vi "Calibration Main.vi"(8 "error in (no error)":errorcluster, 11 "Pump Calibration Config in":T1={"Settings"={"Cycle Period"=500.0, "Ismatech"={"VISA resource name"="", "Simulated?"=TRUE, "Pump Number"=1.0, "Reverse?"=FALSE}, "Masterflex"={"VISA resource name"="", "Simulated?"=TRUE, "Pump Number"=1.0, "Reverse?"=FALSE}, "Bronkhorst M13 Settings"={"VISA resource name"="", "Simulated?"=TRUE, "Smoothing Steps"=1}, "PID 2 Parameters"={"Input Device"=enum."Default", "Output Device"=enum."Default"}, "Tacmina Settings"={"Analog DAQ Task"="", "Digital DAQ Task"=""}, "KNF SIMDOS Settings"={"VISA resource name"="", "Simulated?"=TRUE}, "VICI M50 Settings"={"VISA resource name"="", "Pump ID"="", "Pump Head Vol"=0.0, "Reverse?"=FALSE, "Simulated?"=TRUE}, "FLOM Settings"={"VISA resource name"="", "Simulated?"=TRUE, "Pump Number"=0.0}, "Calibration Limits"={"Minimum (ml/min)"=0.0, "Maximum (ml/min)"=0.0, "Steps"=0.0}, "SSI PR Settings"={"VISA resource name"="", "Simulated?"=FALSE}, "Ismatech 4308 Settings"={"VISA resource name"="", "Pump Number"=1, "Channel Number"=0, "Simulated?"=TRUE, "Reverse?"=FALSE}, "Bronkhorst M14 Settings"={"VISA resource name"="", "Simulated?"=FALSE, "Smoothing Steps"=1}}, "Flowmeter Output"=0.0, "Density"=0.0, "FL Temp"=0.0, "Speed %"=0.0, "File Refnum"=refnum, "Pump On?"=enum."Not Initialized"} {"Settings"."Bronkhorst M14 Settings"."Smoothing Steps" min=1 step=1; "Settings"."Ismatech 4308 Settings"."Channel Number" min=0 max=3; "Settings"."Ismatech 4308 Settings"."Pump Number" min=1; "Settings"."Bronkhorst M13 Settings"."Smoothing Steps" min=1 step=1; "Settings"."Masterflex"."Pump Number" min=1.0 max=20.0 step=1.0; "Settings"."Ismatech"."Pump Number" min=1.0 max=20.0 step=1.0}) -> (0 "error out":errorcluster, 3 "Pump Calibration Config out":T1={"Settings"={"Cycle Period"=500.0, "Ismatech"={"VISA resource name"="", "Simulated?"=TRUE, "Pump Number"=1.0, "Reverse?"=FALSE}, "Masterflex"={"VISA resource name"="", "Simulated?"=TRUE, "Pump Number"=1.0, "Reverse?"=FALSE}, "Bronkhorst M13 Settings"={"VISA resource name"="", "Simulated?"=TRUE, "Smoothing Steps"=1}, "PID 2 Parameters"={"Input Device"=enum."Default", "Output Device"=enum."Default"}, "Tacmina Settings"={"Analog DAQ Task"="", "Digital DAQ Task"=""}, "KNF SIMDOS Settings"={"VISA resource name"="", "Simulated?"=TRUE}, "VICI M50 Settings"={"VISA resource name"="", "Pump ID"="", "Pump Head Vol"=0.0, "Reverse?"=FALSE, "Simulated?"=TRUE}, "FLOM Settings"={"VISA resource name"="", "Simulated?"=TRUE, "Pump Number"=0.0}, "Calibration Limits"={"Minimum (ml/min)"=0.0, "Maximum (ml/min)"=0.0, "Steps"=0.0}, "SSI PR Settings"={"VISA resource name"="", "Simulated?"=FALSE}, "Ismatech 4308 Settings"={"VISA resource name"="", "Pump Number"=1, "Channel Number"=0, "Simulated?"=TRUE, "Reverse?"=FALSE}, "Bronkhorst M14 Settings"={"VISA resource name"="", "Simulated?"=FALSE, "Smoothing Steps"=1}}, "Flowmeter Output"=0.0, "Density"=0.0, "FL Temp"=0.0, "Speed %"=0.0, "File Refnum"=refnum, "Pump On?"=enum."Not Initialized"} {"Settings"."Bronkhorst M14 Settings"."Smoothing Steps" min=1 step=1; "Settings"."Ismatech 4308 Settings"."Channel Number" min=0 max=3; "Settings"."Ismatech 4308 Settings"."Pump Number" min=1; "Settings"."Bronkhorst M13 Settings"."Smoothing Steps" min=1 step=1; "Settings"."Masterflex"."Pump Number" min=1.0 max=20.0 step=1.0; "Settings"."Ismatech"."Pump Number" min=1.0 max=20.0 step=1.0})   [LabVIEW 2018, in "Calibration.lvlib"]
uses:
  Pfizer Timed Seq/Software/Calibration VIs/Calibration.lvlib
  Pump Calibration Config.ctl
  Pfizer Timed Seq/Software/Ismatec ISM 831C/Controls/Ismatech ISM831C Settings Cluster.ctl
  Pfizer Timed Seq/Software/Masterflex 7550-30/Controls/Settings Cluster.ctl
  Pfizer Timed Seq/Software/Bronkhorst M13 Flow Meter/Settings Cluster.ctl
  Pfizer Timed Seq/Software/Measure Instrument/PID Input Enum.ctl
  Pfizer Timed Seq/Software/Measure Instrument/PID 2 Output Enum.ctl
  Pfizer Timed Seq/Software/Tacmina QI/Tacmina QI DAQ Setting.ctl
  Pfizer Timed Seq/Software/KNF Pump/Settings Cluster plus SIMDOS.ctl
  Pfizer Timed Seq/Software/VICI M50 Party Mode/Settings Cluster.ctl
  Pfizer Timed Seq/Software/FLOM Pump/Settings Cluster.ctl
  Pfizer Timed Seq/Software/SSI PR Class/SSI PR or LD Settings Cluster.ctl
  Pfizer Timed Seq/Software/Ismatec 78001/Ismatec 4083.ctl
  Pfizer Timed Seq/Software/Bronkhorst M14 Flow Meter/Settings Cluster.ctl
  Pfizer Timed Seq/Software/Mettler Toledo/Controls/Settings Cluster.ctl
  Pfizer Timed Seq/Software/ASIA Pump/Pump Settings.ctl
  Pfizer Timed Seq/Software/Masterflex 75211/Masterflex 75211 DAQ Setting.ctl
  <vilib>/Platform/TimedLoop/XDataNode/timing_clust.ctl
  <vilib>/Platform/TimedLoop/XDataNode/nitl_modes.ctl
  <vilib>/Platform/TimedLoop/XDataNode/wakeup.ctl
  Pfizer Timed Seq/Software/support/Message Queue/Enqueue Message (Single).vi
  <vilib>/Utility/file.llb/Read Delimited Spreadsheet (string).vi
  <vilib>/Utility/file.llb/Write Delimited Spreadsheet (string).vi
  <vilib>/Platform/TimedLoop/XDataNode/XDataNode.xnode
  <vilib>/regexp/Match Regular Expression.xnode
  Pfizer Timed Seq/Software/KNF Pump/KNF SIMDOS.lvlib
  Pfizer Timed Seq/Software/Ismatec ISM 831C/Ismatec ISM 831C.lvlib
  Pfizer Timed Seq/Software/VICI M50 Party Mode/VICI M6 M50 Party Mode.lvlib
  Pfizer Timed Seq/Software/Masterflex 7550-30/Masterflex 7550-30.lvlib
  Pfizer Timed Seq/Software/FLOM Pump/FLOM Pump.lvlib
  Pfizer Timed Seq/Software/Bronkhorst M13 Flow Meter/Bronkhorst M13 Flow Meter.lvlib
  Pfizer Timed Seq/Software/Bronkhorst M14 Flow Meter/Bronkhorst M14 Flow Meter.lvlib
  Pfizer Timed Seq/Software/support/Message Queue/Message Queue.lvlib
  Pfizer Timed Seq/Software/SSI PR Class/SSI PR or LD Pump.lvlib
  Support/Engine.lvlib
  <vilib>/Analysis/NI_AALPro.lvlib
  <vilib>/Platform/TimedLoop/XDataNode/XDNodeRunTimeDep.lvlib
  Pfizer Timed Seq/Software/Ismatec 78001/Ismatec 4308.lvlib
  Pfizer Timed Seq/Software/Report Generation/Report Generation.lvlib
  Pfizer Timed Seq/Software/Mettler Toledo/Mettler Toledo.lvlib
  Pfizer Timed Seq/Software/Tacmina QI/Tacmina QI.lvlib
  Pfizer Timed Seq/Software/ASIA Pump.lvlib
  Pfizer Timed Seq/Software/Masterflex 75211/Masterflex 75211.lvlib
panel:
  out "Channel Number":i16
  out "Pump Number":i16
  out "Not Empty":bool
  out "All Good":bool
  out "Y array":dbl[](array[numeric])
  out "X array":dbl[](array[numeric])
  out "Output Selected":bool
  out "Input Selected":bool
  out "Step Array":dbl[](array[numeric])
  in  "?":enum32{"Settings", "Results"}(tab)
  in  "Settings Dialog":T17={"Cycle Period"=500.0, "Ismatech"={"VISA resource name"="", "Simulated?"=FALSE, "Pump Number"=1.0, "Reverse?"=FALSE}, "Masterflex"={"VISA resource name"="", "Simulated?"=FALSE, "Pump Number"=1.0, "Reverse?"=FALSE}, "Mettler"={"VISA resource name"="", "Simulated?"=FALSE}, "Bronkhorst M13 Flow Meter"={"VISA resource name"="", "Simulated?"=FALSE, "Smoothing Steps"=1}, "Setup Parameters"={"Input Device"=enum."Default", "Output Device"=enum."Default"}, "Bronkhorst M14 Settings"={"VISA resource name"="", "Simulated?"=FALSE, "Smoothing Steps"=1}, "Tacmina Settings"={"Analog DAQ Task"="", "Digital DAQ Task"=""}, "KNF SIMDOS Settings"={"VISA resource name"="", "Simulated?"=FALSE}, "ASIA Pump C"={"ASIA Pump #"=-1, "channel"=-1, "Simulated"=FALSE}, "VICI M50 Settings"={"VISA resource name"="", "Pump ID"="", "Pump Head Vol"=0.0, "Reverse?"=FALSE, "Simulated?"=FALSE}, "FLOM Settings"={"VISA resource name"="", "Simulated?"=FALSE, "Pump Number"=1.0}, "Calibration Limits"={"Minimum (ml/min)"=0.0, "Maximum (ml/min)"=0.0, "Steps"=0.0}, "File Name"="", "SSI PR Settings"={"VISA resource name"="", "Simulated?"=FALSE}, "Masterflex 75211 Settings"={"Analog DAQ Task"="", "Digital DAQ Task"=""}, "Ismatech 4308 Settings"={"VISA resource name"="", "Pump Number"=0, "Channel Number"=0, "Simulated?"=FALSE, "Reverse?"=FALSE}} {"Ismatech 4308 Settings"."Channel Number" min=0 max=3; "Ismatech 4308 Settings"."Pump Number" min=1; "Calibration Limits"."Maximum (ml/min)" max=16.5; "ASIA Pump C"."channel" min=-1 max=1 step=1; "Bronkhorst M14 Settings"."Smoothing Steps" min=1 step=1; "Bronkhorst M13 Flow Meter"."Smoothing Steps" min=1 step=1; "Masterflex"."Pump Number" min=1.0 max=20.0 step=1.0; "Ismatech"."Pump Number" min=1.0 max=20.0 step=1.0}
  in  "Start Button":bool
  in  "Cancel Button":bool
  out "Y Intercept":dbl
  in  "Accept Button":bool
  in  "Decline Button":bool
  out "Calibration Graph":cluster{dbl[], dbl[]}[](graph)
  out "Calibration Slope":dbl
  out "R^2 Value":dbl format="%#.4g"
  out "Pump Status":enum16{"Off", "On", "Not Initialized"}(ring)
  # "Output Instruments"
  # "Input Instruments"
  # "Output Instruments"
  # "Input Instruments"
  # "Output Instruments"
  # "Input Instruments"
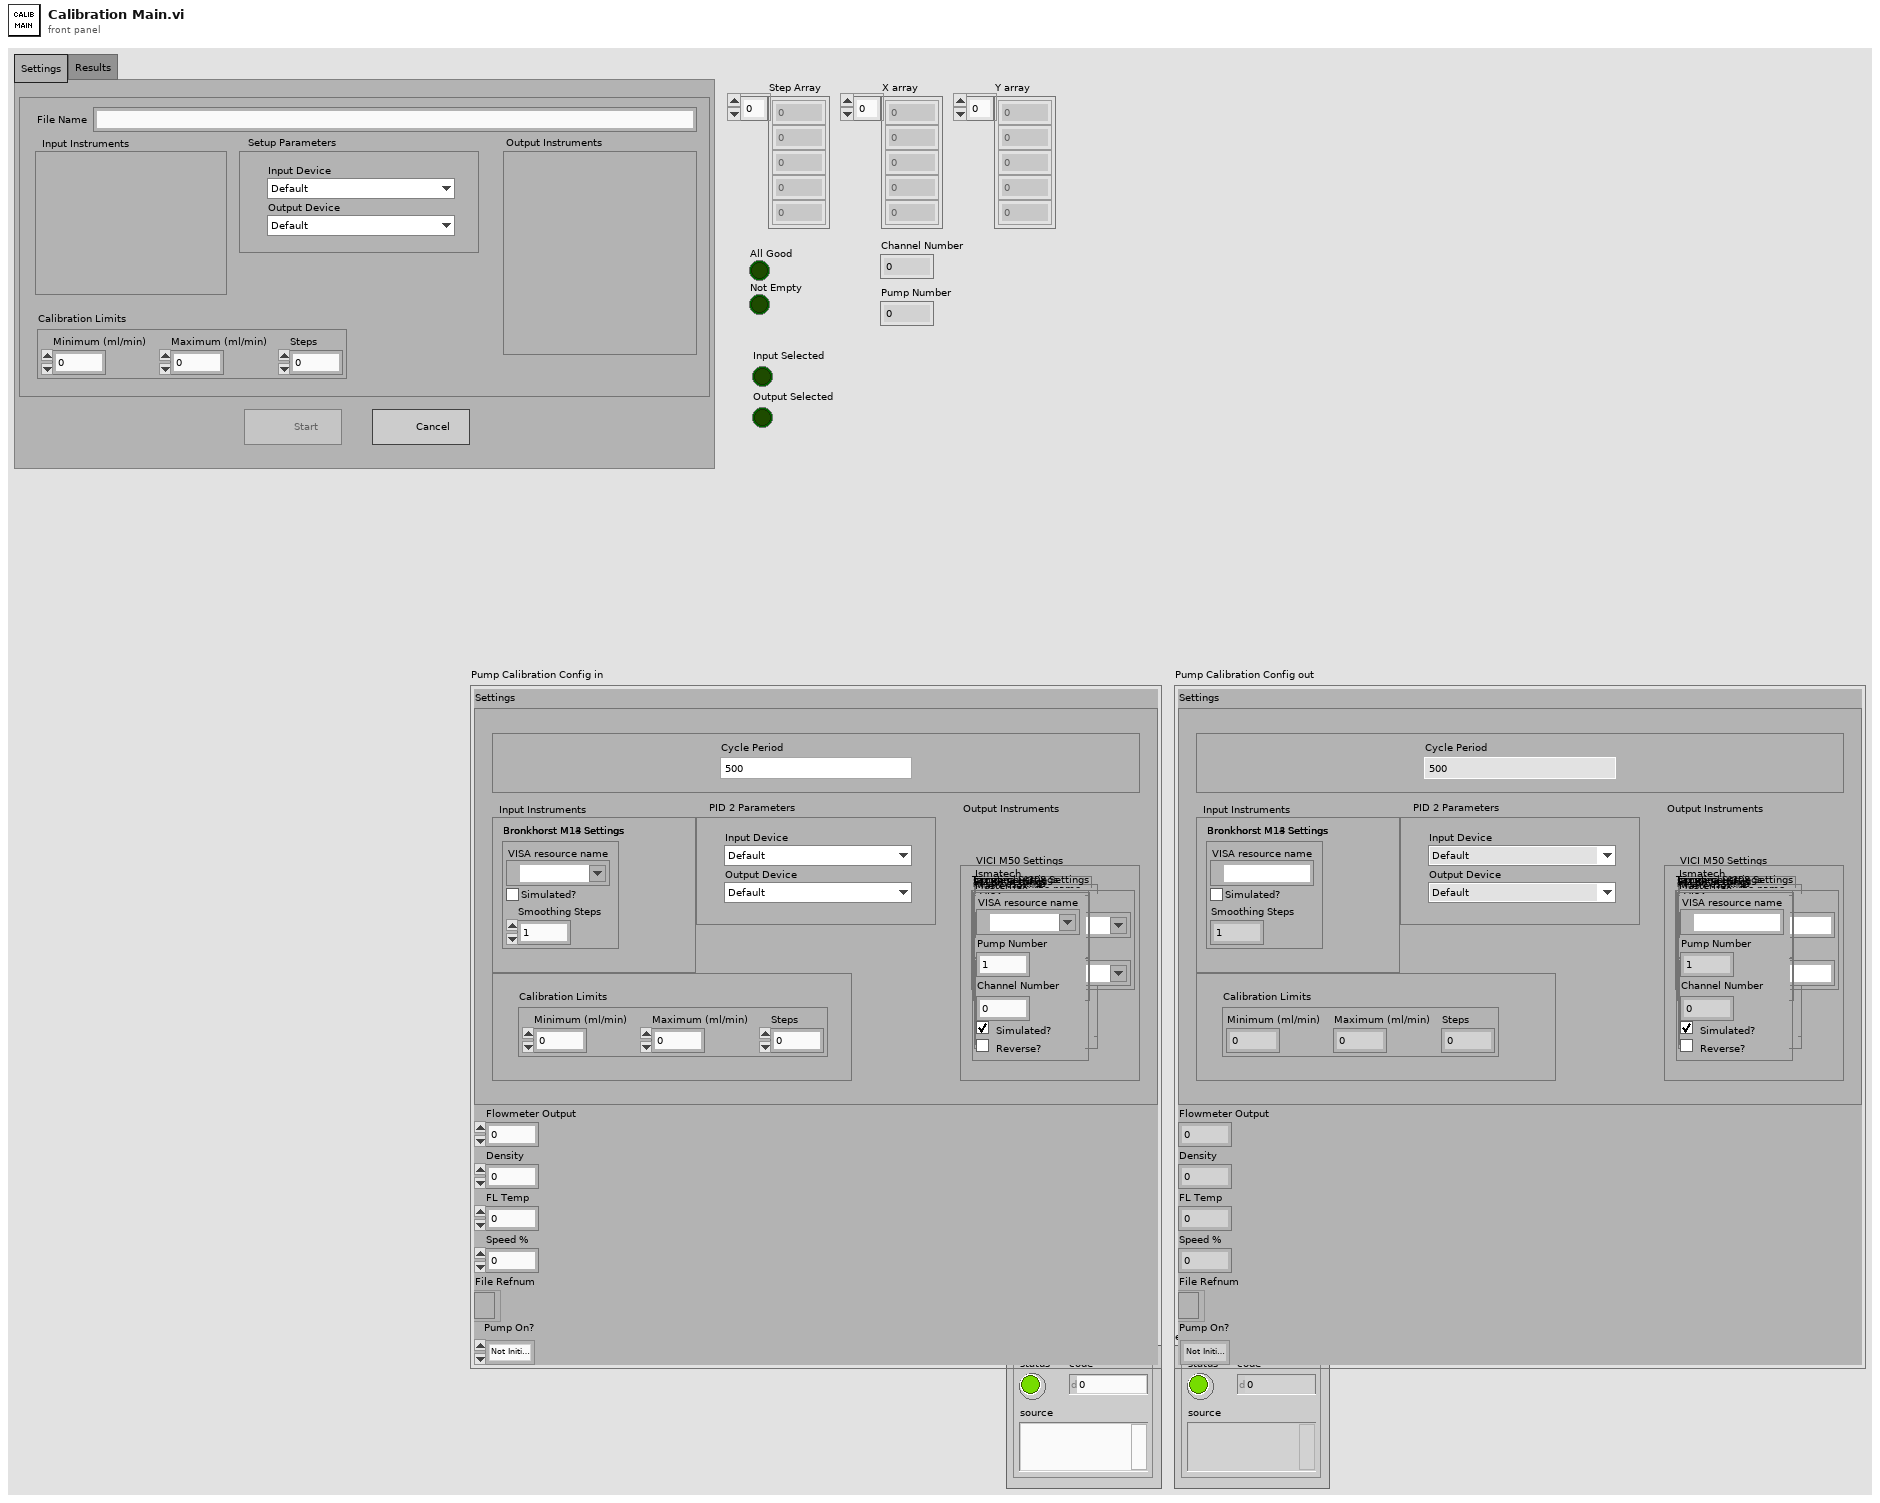
[diagram p1: front panel]
types:
  T1 = typedef "Calibration.lvlib/Pump Calibration Config.ctl" = cluster{"Settings":cluster{"Cycle Period":dbl, "Ismatech":T2, "Masterflex":T3, "Bronkhorst M13 Settings":T4, "PID 2 Parameters":cluster{"Input Device":T5, "Output Device":T6}, "Tacmina Settings":T7, "KNF SIMDOS Settings":T8, "VICI M50 Settings":T9, "FLOM Settings":T10, "Calibration Limits":cluster{"Minimum (ml/min)":dbl, "Maximum (ml/min)":dbl, "Steps":dbl}, "SSI PR Settings":T11, "Ismatech 4308 Settings":T12, "Bronkhorst M14 Settings":T13}, "Flowmeter Output":dbl, "Density":dbl, "FL Temp":dbl, "Speed %":dbl, "File Refnum":refnum<file>, "Pump On?":enum16{"Off", "On", "Not Initialized"}}
  T2 = typedef "Ismatec ISM 831C.lvlib/Ismatech ISM831C Settings Cluster.ctl" = cluster{"VISA resource name":refnum<visa-resource-name>, "Simulated?":bool, "Pump Number":dbl, "Reverse?":bool}
  T3 = typedef "Masterflex 7550-30.lvlib/Settings Cluster.ctl" = cluster{"VISA resource name":refnum<visa-resource-name>, "Simulated?":bool, "Pump Number":dbl, "Reverse?":bool}
  T4 = typedef "Bronkhorst M13 Flow Meter.lvlib/Settings Cluster.ctl" = cluster{"VISA resource name":refnum<visa-resource-name>, "Simulated?":bool, "Smoothing Steps":i32}
  T5 = typedef "PID Input Enum.ctl" = enum16{"Default", "Bronkhorst M13", "Bronkhorst M14", "Scale Rate of Change"}
  T6 = typedef "PID 2 Output Enum.ctl" = enum16{"Default", "Ismatec ISM 4308", "Ismatec ISM 831C", "Masterflex 7550-30", "VICI M6", "VICI M50", "Tacmina QI", "KNF SIMDOS", "ASIA Type C", "FLOM UI-22-11", "SSI PR/LD", "SSI P40", "Masterflex 75211-70"}
  T7 = typedef "Tacmina QI.lvlib/Tacmina QI DAQ Setting.ctl" = cluster{"Analog DAQ Task":refnum<k21>, "Digital DAQ Task":refnum<k21>}
  T8 = typedef "KNF SIMDOS.lvlib/Settings Cluster plus SIMDOS.ctl" = cluster{"VISA resource name":refnum<visa-resource-name>, "Simulated?":bool}
  T9 = typedef "VICI M6 M50 Party Mode.lvlib/Settings Cluster.ctl" = cluster{"VISA resource name":refnum<visa-resource-name>, "Pump ID":string, "Pump Head Vol":dbl, "Reverse?":bool, "Simulated?":bool}
  T10 = typedef "FLOM Pump.lvlib/Settings Cluster.ctl" = cluster{"VISA resource name":refnum<visa-resource-name>, "Simulated?":bool, "Pump Number":dbl}
  T11 = typedef "SSI PR or LD Pump.lvlib/SSI PR or LD Settings Cluster.ctl" = cluster{"VISA resource name":refnum<visa-resource-name>, "Simulated?":bool}
  T12 = typedef "Ismatec 4308.lvlib/Ismatec 4083.ctl" = cluster{"VISA resource name":refnum<visa-resource-name>, "Pump Number":i16, "Channel Number":i16, "Simulated?":bool, "Reverse?":bool}
  T13 = typedef "Bronkhorst M14 Flow Meter.lvlib/Settings Cluster.ctl" = cluster{"VISA resource name":refnum<visa-resource-name>, "Simulated?":bool, "Smoothing Steps":i32}
  T14 = typedef "Mettler Toledo.lvlib/Settings Cluster.ctl" = cluster{"VISA resource name":refnum<visa-resource-name>, "Simulated?":bool}
  T15 = typedef "ASIA Pump.lvlib/Pump Settings.ctl" = cluster{"ASIA Pump #":i32, "channel":i32, "Simulated":bool}
  T16 = typedef "Masterflex 75211.lvlib/Masterflex 75211 DAQ Setting.ctl" = cluster{"Analog DAQ Task":refnum<k21>, "Digital DAQ Task":refnum<k21>}
  T17 = cluster{"Cycle Period":dbl, "Ismatech":T2, "Masterflex":T3, "Mettler":T14, "Bronkhorst M13 Flow Meter":T4, "Setup Parameters":cluster{"Input Device":T5, "Output Device":T6}, "Bronkhorst M14 Settings":T13, "Tacmina Settings":T7, "KNF SIMDOS Settings":T8, "ASIA Pump C":T15, "VICI M50 Settings":T9, "FLOM Settings":T10, "Calibration Limits":cluster{"Minimum (ml/min)":dbl, "Maximum (ml/min)":dbl, "Steps":dbl}, "File Name":string, "SSI PR Settings":T11, "Masterflex 75211 Settings":T16, "Ismatech 4308 Settings":T12}
  T18 = enum8{"Enabled", "Disabled", "Disabled and Grayed Out"}
  T19 = cluster{"Calibration UI":refnum<queue>, "Calibration Engine":refnum<queue>}
  T20 = typedef "XDNodeRunTimeDep.lvlib/timing_clust.ctl" = cluster{"Expected End [f-1]":u64, "Actual End [f-1]":u64, "Finished Late? [f-1]":bool, "Expected End [i-1]":u64, "Actual End [i-1]":u64, "Finished Late? [i-1]":bool, "Expected Start [i]":u64, "Actual Start [i]":u64, "Expected Start [f]":u64, "Actual Start [f]":u64, "Source Name":string, "Structure Name":string, "Period":i64, "Deadline":i64, "Offset":i64, "Start":i64, "Priority":i32, "Timeout":i32, "Mode":T21, "Wakeup Reason":T22, "Error":errorcluster, "Source Type":string, "Secondary Source Type":string, "Global End Time":u64, "Global Start Time":u64, "Frame Duration":u64, "Iteration Duration":u64, "Assigned CPU":i32, "I/O Scan Engine Mode":u32}
  T21 = typedef "XDNodeRunTimeDep.lvlib/nitl_modes.ctl" = enum32{"No Change", "Process missed periods, maintain original phase", "Discard missed periods, maintain original phase", "Process missed periods, ignore original phase", "Discard missed periods, ignore original phase"}
  T22 = typedef "XDNodeRunTimeDep.lvlib/wakeup.ctl" = enum32{"Normal", "Aborted", "Asynchronous wakeup", "Timing source error", "Timed loop error", "Timeout"}
  T23 = enum16{"open", "replace", "create", "open or create", "replace or create", "replace or create with confirmation"}
  T24 = cluster{"R^2":dbl, "Calibration Slope":dbl, "Y Intercept":dbl}
  T25 = cluster{"slope min":dbl, "slope max":dbl, "intercept min":dbl, "intercept max":dbl}
  T26 = cluster{"Minimum (ml/min)":dbl, "Maximum (ml/min)":dbl, "Steps":dbl}
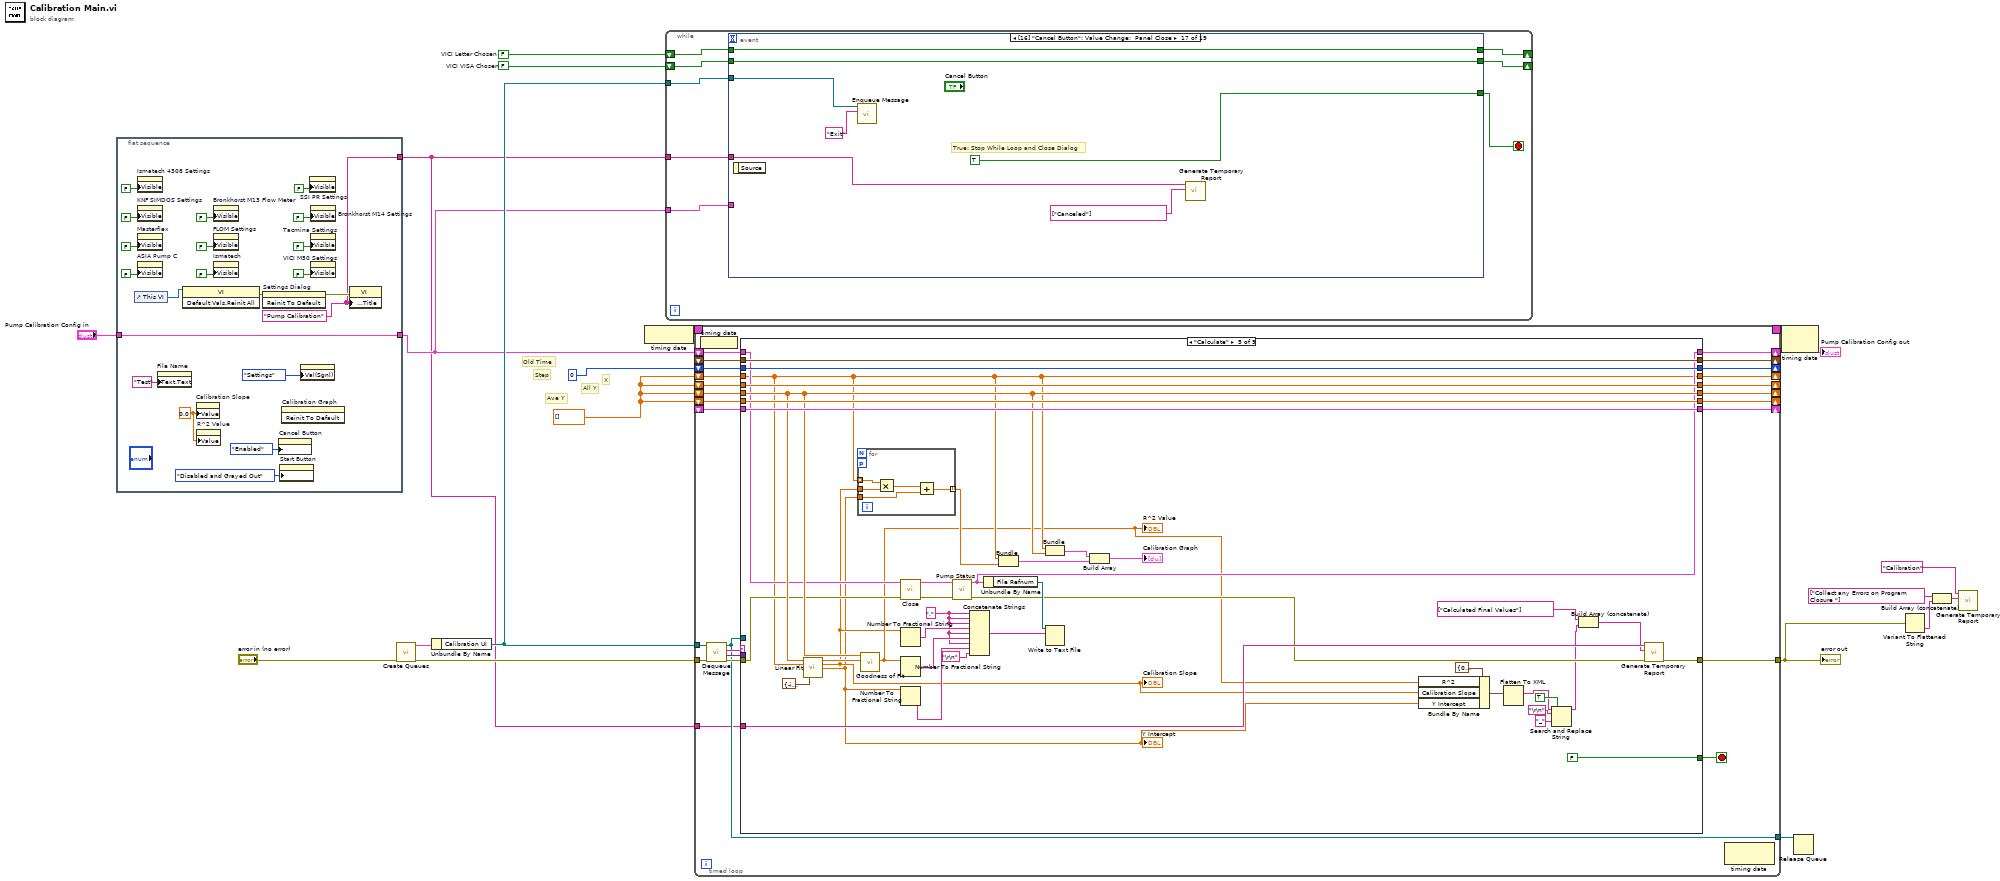
[diagram p0: block diagram]
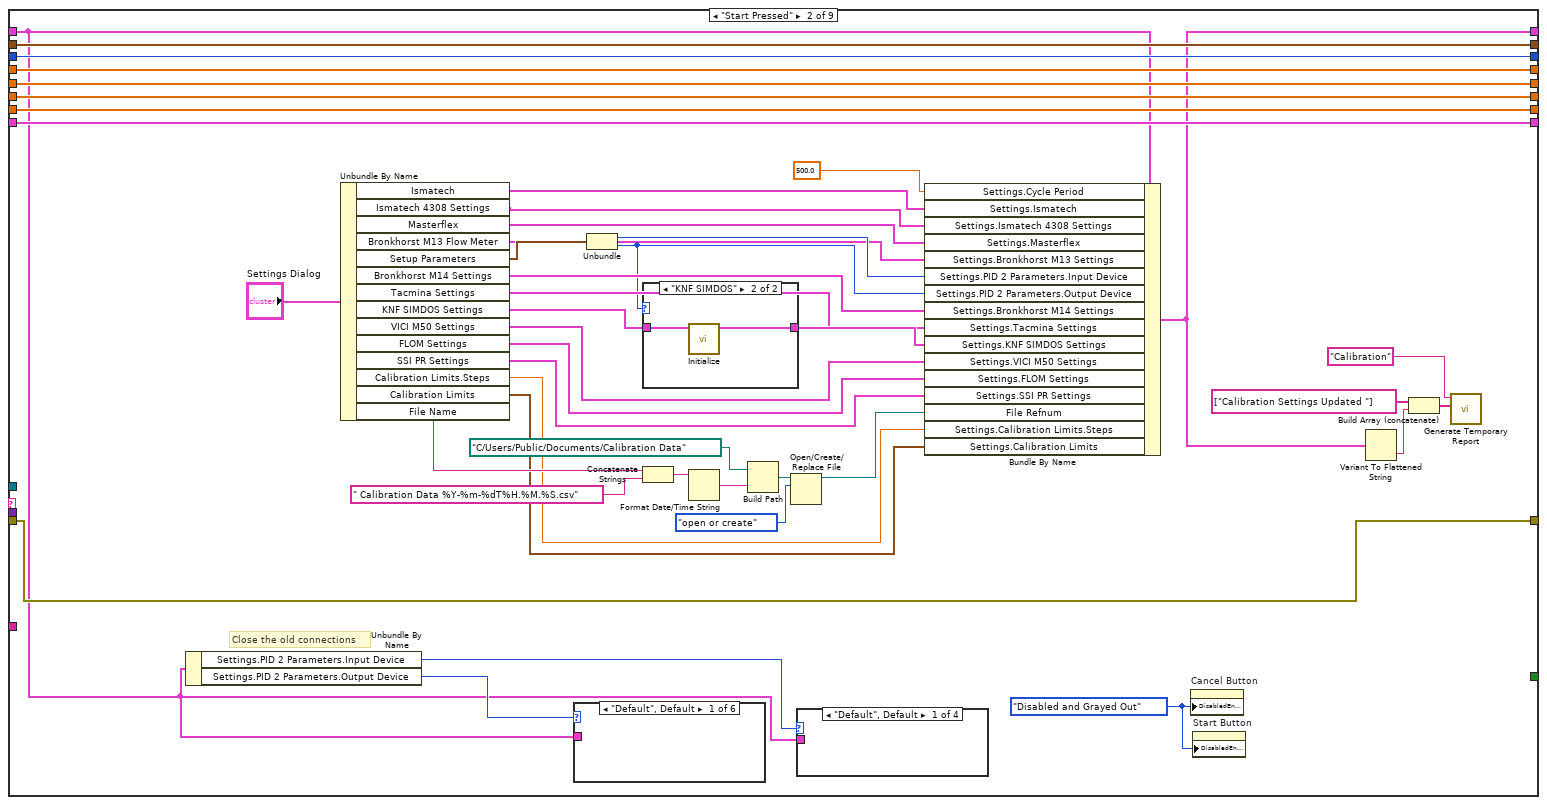
[diagram p3: hidden frame]
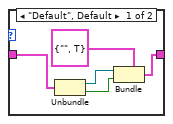
[diagram p4: hidden frame]
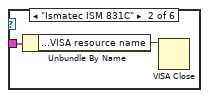
[diagram p5: hidden frame]
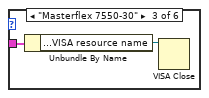
[diagram p6: hidden frame]
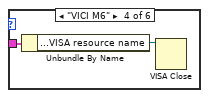
[diagram p7: hidden frame]
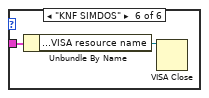
[diagram p9: hidden frame]
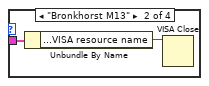
[diagram p10: hidden frame]
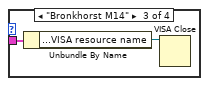
[diagram p11: hidden frame]
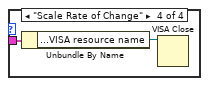
[diagram p12: hidden frame]
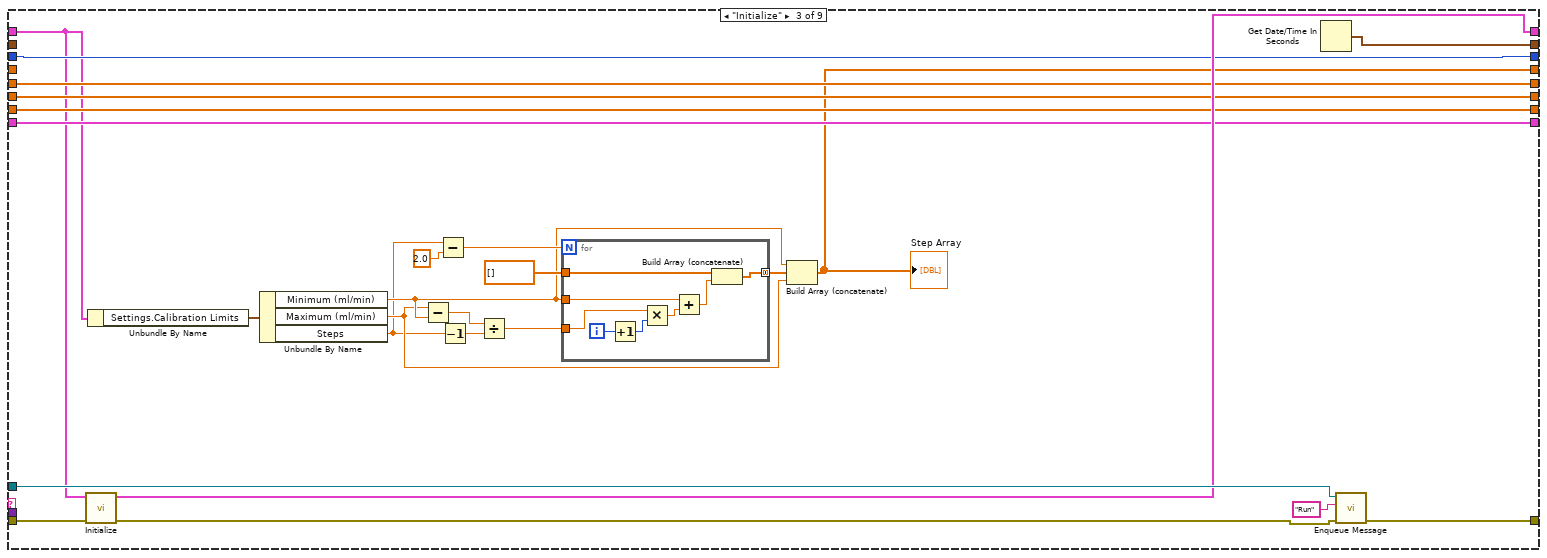
[diagram p13: hidden frame]
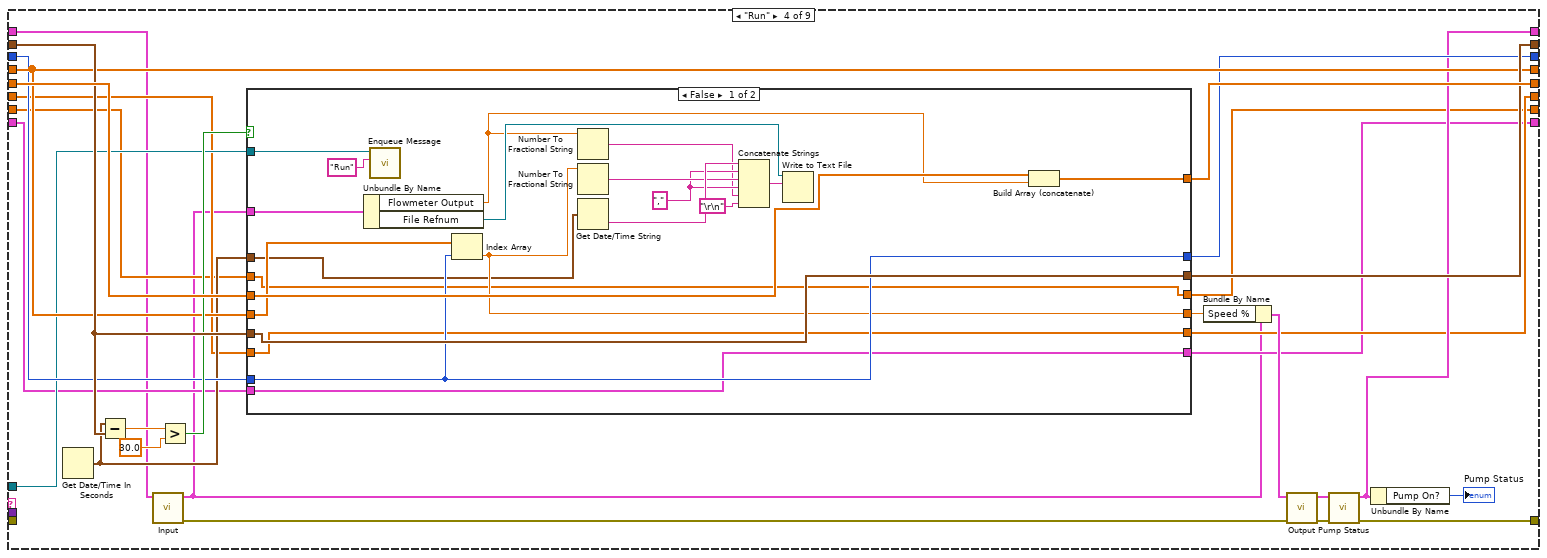
[diagram p14: hidden frame]
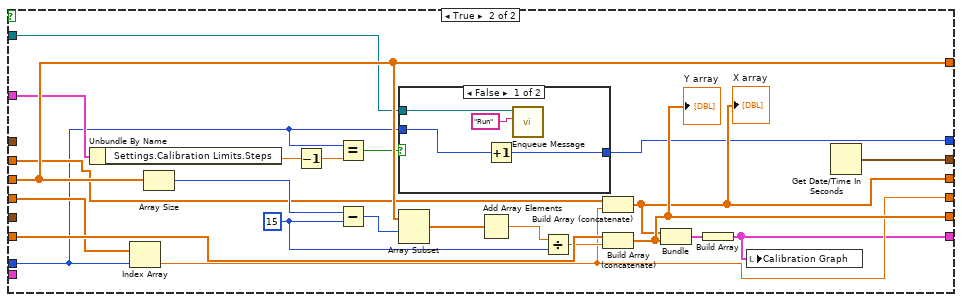
[diagram p15: hidden frame]
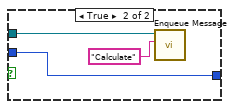
[diagram p16: hidden frame]
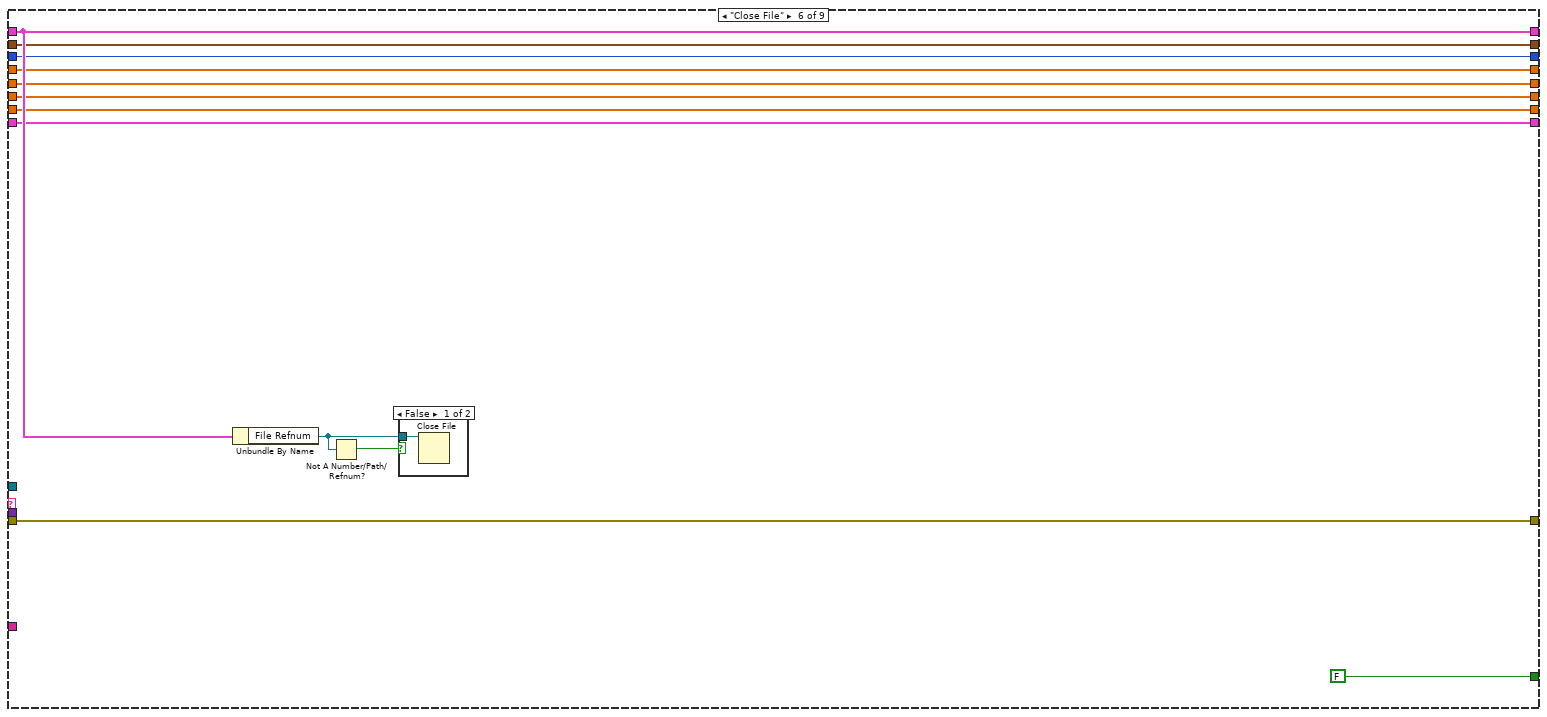
[diagram p17: hidden frame]
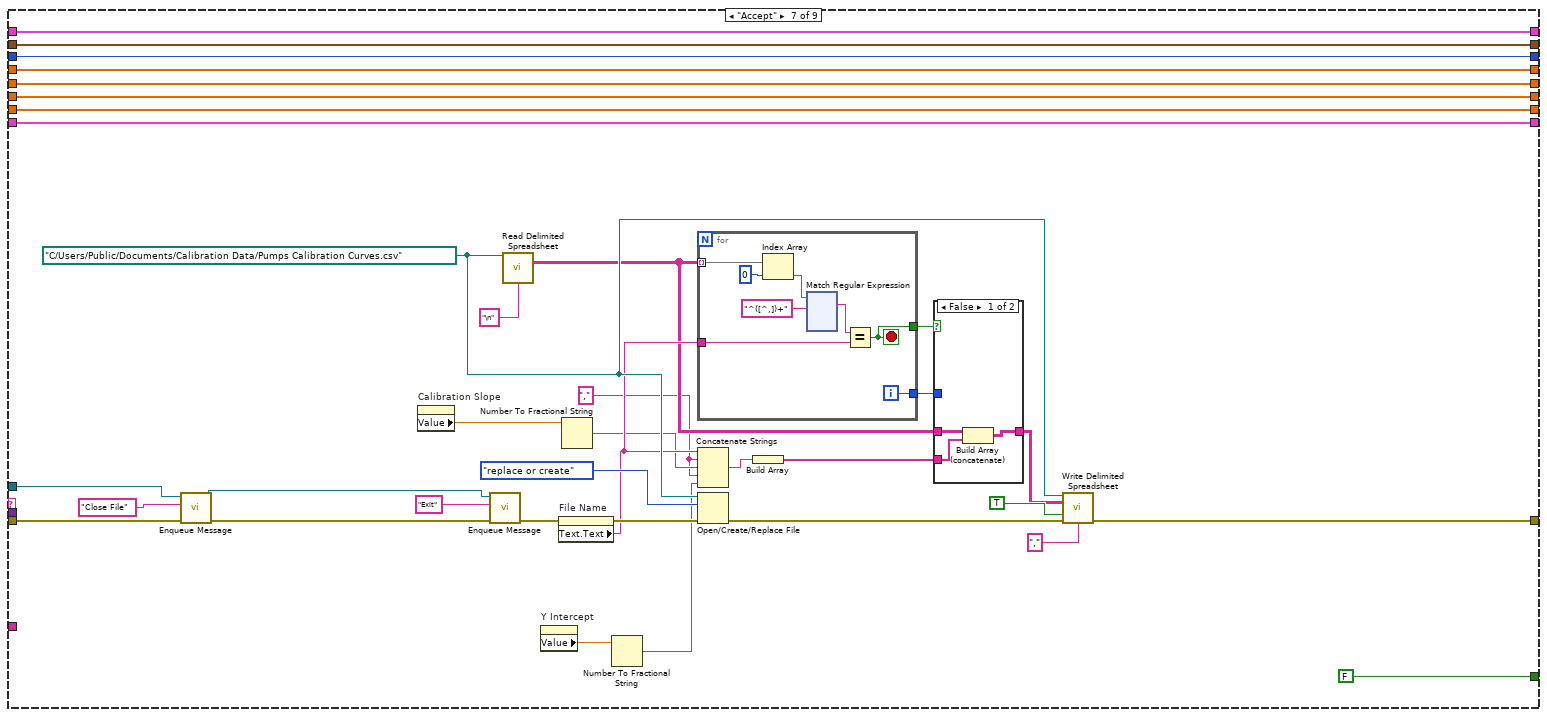
[diagram p19: hidden frame]
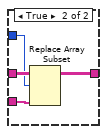
[diagram p20: hidden frame]
diagram:
  w8 = dbl[] []
  w19 = FALSE  # VICI VISA Chosen
  w20 = FALSE  # VICI Letter Chosen
  # "Old Time"
  # "Step"
  # "Ave Y"
  # "All Y"
  # "X"
  n1 = flat-sequence {
    tunnel: "Pump Calibration Config in" -> [w41]
    tunnel: [w41] -> w14
    tunnel: [w21] -> w1
    frame #0 {
      w38 = 0.0 ("Calibration Slope")
      w21 = "Pump Calibration" ("string")
      n2 = control-ref of="This VI"() -> (w37:refnum<vi>)
      n3 = property on="Ismatech 4308 Settings" class="Clust (strict)"("Visible"=FALSE) -> ()  [unwired: 2 in, 2 out]
      n4 = property on="KNF SIMDOS Settings" class="Clust (strict)"("Visible"=FALSE) -> ()  [unwired: 2 in, 2 out]
      n5 = property on="Masterflex" class="Clust (strict)"("Visible"=FALSE) -> ()  [unwired: 2 in, 2 out]
      n6 = property on="ASIA Pump C" class="Clust (strict)"("Visible"=FALSE) -> ()  [unwired: 2 in, 2 out]
      n7 = property on="File Name" class="Str"("Text.Text"="Test") -> ()  [unwired: 2 in, 2 out]
      n8 = invoke class="VI" method="Default Vals.Reinit All"(reference=w37) -> (error out=w23:errorcluster)  [unwired: 2 in, 2 out]
      n9 = property on="Calibration Slope" class="DigNum (strict)"("Value"=w38) -> ()  [unwired: 2 in, 2 out]
      n10 = property on="R^2 Value" class="DigNum (strict)"("Value"=w38) -> ()  [unwired: 2 in, 2 out]
      n11 = property on="Bronkhorst M13 Flow Meter" class="Clust (strict)"("Visible"=FALSE) -> ()  [unwired: 2 in, 2 out]
      n12 = property on="FLOM Settings" class="Clust (strict)"("Visible"=FALSE) -> ()  [unwired: 2 in, 2 out]
      n13 = property on="Ismatech" class="Clust (strict)"("Visible"=FALSE) -> ()  [unwired: 2 in, 2 out]
      n14 = invoke on="Settings Dialog" class="Clust (strict)" method="Reinit To Default"(error in=w23) -> (error out=w22:errorcluster)  [unwired: 2 in, 2 out]
      n15 = property on="Cancel Button" class="Bool"("DisabledEnum"=T18."Enabled" ("Disabled")) -> ()  [unwired: 2 in, 2 out]
      n16 = property on="Start Button" class="Bool"("DisabledEnum"=T18."Disabled and Grayed Out" ("Disabled")) -> ()  [unwired: 2 in, 2 out]
      n17 = invoke on="Calibration Graph" class="XYGraph (strict)" method="Reinit To Default"() -> ()  [unwired: 3 in, 3 out]
      n18 = property class="TabCtl (strict)"("Val(Sgnl)"=enum32{"Settings", "Results"}."Settings") -> ()  [unwired: 2 in, 2 out]
      n19 = property on="SSI PR Settings" class="Clust (strict)"("Visible"=FALSE) -> ()  [unwired: 2 in, 2 out]
      n20 = property on="Bronkhorst M14 Settings" class="Clust (strict)"("Visible"=FALSE) -> ()  [unwired: 2 in, 2 out]
      n21 = property on="Tacmina Settings" class="Clust (strict)"("Visible"=FALSE) -> ()  [unwired: 2 in, 2 out]
      n22 = property on="VICI M50 Settings" class="Clust (strict)"("Visible"=FALSE) -> ()  [unwired: 2 in, 2 out]
      n23 = property class="VI"(error in=w22, "Front Panel.Title"=w21) -> ()  [unwired: 1 in, 2 out]
    }
  }
  n24 = call "Create Queues.vi"("error in (no error)"="error in (no error)") -> ("error out"=w13:errorcluster, "Message Queues Out"=w16:T19)  [unwired: 9 in]
  n25 = Unbundle By Name(w16) -> ("Calibration UI"=w15:refnum<queue>)
  n26 = node-c288() -> (w11:T20)
  n27 = while {
    shift-right: [w48] -> _
    shift-left: w20 -> [w47]
    shift-right: [w46] -> _
    shift-left: w19 -> [w45]
    tunnel: w14 -> [w43]
    tunnel: w15 -> [w44]
    tunnel: w1 -> [w42]
    stop <- w49 stop-if-true
    n28 = event shown="[16] \"Cancel Button\": Value Change;  Panel Close" {
      selector: _ -> [_ _ _ _ _ _ _ _ _ _ _ _ _ _ _ _ _ _ _]
      dyn-events: _ -> [_ _ _ _ _ _ _ _ _ _ _ _ _ _ _ _ _ _ _]
      timeout: _ -> [_ _ _ _ _ _ _ _ _ _ _ _ _ _ _ _ _ _ _]
      tunnel: [FALSE _ _ _ _ _ _ _ _ _ _ _ _ _ _ _ TRUE TRUE TRUE] -> w49
      tunnel: [w58 w61 w87 w102 TRUE w129 w134 w147 w164 w182 w197 w208 w212 w226 w241 w260 w373 w380 w387] -> w48
      tunnel: w47 -> [w58 w61 w87 w102 _ w129 w134 w147 w164 w182 w197 w208 w212 w226 w241 w260 w373 w380 w387]
      tunnel: [w57 w60 w86 TRUE w117 w132 w133 w146 w163 w181 w196 w207 w211 w225 w240 w259 w372 w379 w386] -> w46
      tunnel: w45 -> [w57 w60 w86 _ w117 w132 w133 w146 w163 w181 w196 w207 w211 w225 w240 w259 w372 w379 w386]
      tunnel: w44 -> [w53 _ _ _ _ _ _ _ _ _ _ _ _ _ _ _ w370 w377 w384]
      tunnel: w43 -> [_ _ _ _ _ _ _ _ _ _ _ _ _ _ w239 w258 _ _ _]
      tunnel: w42 -> [w50 _ _ _ _ _ _ _ _ _ _ _ _ _ _ _ w368 w375 w382]
      event "Start Button": Value Change {
        n29 = event-data() -> ()  [unwired: 1 in, 1 out]
        n30 = call-poly "Enqueue Message.vi"("Message"="Start Pressed", "Message Queue"=w53) -> ("dup Message Queue"=w52:refnum<queue>)  [unwired: 8 in, 1 out]
        n31 = property class="TabCtl (strict)"("Val(Sgnl)"=enum32{"Settings", "Results"}."Results") -> ()  [unwired: 2 in, 2 out]
        n32 = call-poly "Enqueue Message.vi"("Message"="Initialize", "Message Queue"=w52) -> ()  [unwired: 8 in, 2 out]
        n33 = call "Generate Temporary Report.vi"("Line of Events"=string[] ["Started"], "Module Name"=w50) -> ()  [unwired: 9 in, 1 out]
      }
      event Value Change {
        n34 = event-data() -> ("OldVal"=w63:refnum<visa-resource-name>)  [unwired: 1 in]
        n35 = local read "Settings Dialog"() -> (w66:T17)
        n36 = VISA Close(VISA resource name=w63) -> (error out=w64:errorcluster)  [unwired: 1 in]
        n37 = Unbundle By Name(w66) -> ("Ismatech"=w65:T2)
        n38 = call "Initialize.vi"("error in (no error)"=w64, "Ismatech Settings"=w65) -> ("No Pump Connected"=w62:bool)  [unwired: 6 in, 3 out]
        n39 = case shown="False" w62 {
          frame False {
            n40 = local read "Input Selected"() -> (w68:bool)
            n41 = case shown="True" w68 {
              frame False {
              }
              frame True {
                n42 = control-ref of="Start Button"() -> (w70:refnum<vi>)
                n43 = property on="Property Node" class="Bool"(reference=w70, "DisabledEnum"=T18."Enabled" ("Disabled")) -> ()  [unwired: 1 in, 2 out]
              }
            }
            "Output Selected" <- TRUE ("Output Selected")
          }
          frame True {
            n44 = control-ref of="Start Button"() -> (w71:refnum<vi>)
            n45 = property on="Property Node" class="Bool"(reference=w71, "DisabledEnum"=T18."Disabled and Grayed Out" ("Disabled")) -> ()  [unwired: 1 in, 2 out]
          }
        }
      }
      event Value Change {
        n46 = event-data() -> ("OldVal"=w77:T12, "NewVal"=w85:T12)  [unwired: 1 in]
        n47 = Unbundle By Name(w85) -> ("VISA resource name"=w75:refnum<visa-resource-name>, "Pump Number"=w84:i16, "Channel Number"=w83:i16)
        "Pump Number" <- w84
        "Channel Number" <- w83
        n48 = Unbundle By Name(w77) -> ("VISA resource name"=w76:refnum<visa-resource-name>)
        n49 = Not Equal?(x=w76, y=w75) -> (x != y?=w73:bool)
        n50 = Empty String/Path?(string/path=w75) -> (empty?=w82:bool)
        n51 = case shown="True" w73 {
          tunnel: w76 -> [_ w90]
          tunnel: [errorcluster {"status"=FALSE, "code"=0, "source"=""} ("error out") w89] -> w74
          frame False {
          }
          frame True {
            n52 = VISA Close(VISA resource name=w90) -> (error out=w89:errorcluster)  [unwired: 1 in]
          }
        }
        n53 = Not(x=w82) -> (.not. x?=w81:bool)
        "Not Empty" <- w81
        n54 = Greater Than 0?(x=w84) -> (x > 0?=w80:bool)
        n55 = Greater Than 0?(x=w83) -> (x > 0?=w79:bool)
        n56 = Compound Arithmetic op=AND(w81, w80, w79) -> (w78:bool)
        "All Good" <- w78
        n57 = case shown="True" w78 {
          tunnel: w85 -> [_ w95]
          tunnel: w74 -> [_ w94]
          frame False {
            n58 = control-ref of="Start Button"() -> (w92:refnum<vi>)
            n59 = property on="Property Node" class="Bool"(reference=w92, "DisabledEnum"=T18."Disabled and Grayed Out" ("Disabled")) -> ()  [unwired: 1 in, 2 out]
          }
          frame True {
            n60 = call "Initialize.vi"("error in (no error)"=w94, "Ismatech 3 Channel Settings In"=w95) -> ("Initialized"=w93:bool)  [unwired: 6 in, 3 out]
            n61 = case shown="True" w93 {
              frame False {
                n62 = control-ref of="Start Button"() -> (w96:refnum<vi>)
                n63 = property on="Property Node" class="Bool"(reference=w96, "DisabledEnum"=T18."Disabled and Grayed Out" ("Disabled")) -> ()  [unwired: 1 in, 2 out]
              }
              frame True {
                n64 = local read "Input Selected"() -> (w99:bool)
                n65 = case shown="True" w99 {
                  frame False {
                  }
                  frame True {
                    n66 = control-ref of="Start Button"() -> (w101:refnum<vi>)
                    n67 = property on="Property Node" class="Bool"(reference=w101, "DisabledEnum"=T18."Enabled" ("Disabled")) -> ()  [unwired: 1 in, 2 out]
                  }
                }
                n68 = local write "Output Selected"(TRUE ("Output Selected")) -> ()
              }
            }
          }
        }
      }
      event Value Change {
        n69 = event-data() -> ("OldVal"=w104:refnum<visa-resource-name>)  [unwired: 1 in]
        n70 = local read "Settings Dialog"() -> (w107:T17)
        n71 = Unbundle By Name(w107) -> ("VICI M50 Settings"=w106:T9)
        n72 = VISA Close(VISA resource name=w104) -> (error out=w105:errorcluster)  [unwired: 1 in]
        n73 = case shown="True" w102 {
          tunnel: w106 -> [_ w110]
          tunnel: w105 -> [_ w109]
          frame False {
          }
          frame True {
            n74 = call "Initialize.vi"("error in (no error)"=w109, "VICI Settings"=w110) -> ("No Pump Connected"=w108:bool)  [unwired: 6 in, 3 out]
            n75 = case shown="False" w108 {
              frame False {
                n76 = local read "Input Selected"() -> (w111:bool)
                n77 = case shown="True" w111 {
                  frame False {
                  }
                  frame True {
                    n78 = control-ref of="Start Button"() -> (w114:refnum<vi>)
                    n79 = property on="Property Node" class="Bool"(reference=w114, "DisabledEnum"=T18."Enabled" ("Disabled")) -> ()  [unwired: 1 in, 2 out]
                  }
                }
                n80 = local write "Output Selected"(TRUE) -> ()
              }
              frame True {
                n81 = control-ref of="Start Button"() -> (w115:refnum<vi>)
                n82 = property on="Property Node" class="Bool"(reference=w115, "DisabledEnum"=T18."Disabled and Grayed Out" ("Disabled")) -> ()  [unwired: 1 in, 2 out]
              }
            }
          }
        }
      }
      event Value Change {
        n83 = event-data() -> ()  [unwired: 1 in, 1 out]
        n84 = local read "Settings Dialog"() -> (w120:T17)
        n85 = Unbundle By Name(w120) -> ("VICI M50 Settings"=w119:T9)
        n86 = case shown="True" w117 {
          tunnel: w119 -> [_ w122]
          frame False {
          }
          frame True {
            n87 = call "Initialize.vi"("VICI Settings"=w122) -> ("No Pump Connected"=w121:bool)  [unwired: 7 in, 3 out]
            n88 = case shown="False" w121 {
              frame False {
                n89 = local read "Input Selected"() -> (w123:bool)
                n90 = case shown="True" w123 {
                  frame False {
                  }
                  frame True {
                    n91 = control-ref of="Start Button"() -> (w126:refnum<vi>)
                    n92 = property on="Property Node" class="Bool"(reference=w126, "DisabledEnum"=T18."Enabled" ("Disabled")) -> ()  [unwired: 1 in, 2 out]
                  }
                }
                n93 = local write "Output Selected"(TRUE) -> ()
              }
              frame True {
                n94 = control-ref of="Start Button"() -> (w127:refnum<vi>)
                n95 = property on="Property Node" class="Bool"(reference=w127, "DisabledEnum"=T18."Disabled and Grayed Out" ("Disabled")) -> ()  [unwired: 1 in, 2 out]
              }
            }
          }
        }
      }
      event Value Change {
        n96 = event-data() -> ()  [unwired: 1 in, 6 out]
        n97 = control-ref of="Start Button"() -> (w131:refnum<vi>)
        n98 = property on="Property Node" class="Bool"(reference=w131, "DisabledEnum"=T18."Enabled" ("Disabled")) -> ()  [unwired: 1 in, 2 out]
      }
      event Value Change {
        n99 = event-data() -> ("OldVal"=w136:refnum<visa-resource-name>)  [unwired: 1 in]
        n100 = local read "Settings Dialog"() -> (w138:T17)
        n101 = VISA Close(VISA resource name=w136) -> (error out=w137:errorcluster)  [unwired: 1 in]
        n102 = Unbundle By Name(w138) -> ("Masterflex"=w139:T3)
        n103 = call "Initialize.vi"("error in (no error)"=w137, "Masterflex Settings in"=w139) -> ("No Pump Connected"=w135:bool)  [unwired: 6 in, 3 out]
        n104 = case shown="False" w135 {
          frame False {
            n105 = local read "Input Selected"() -> (w140:bool)
            n106 = case shown="True" w140 {
              frame False {
              }
              frame True {
                n107 = control-ref of="Start Button"() -> (w143:refnum<vi>)
                n108 = property on="Property Node" class="Bool"(reference=w143, "DisabledEnum"=T18."Enabled" ("Disabled")) -> ()  [unwired: 1 in, 2 out]
              }
            }
            n109 = local write "Output Selected"(TRUE) -> ()
          }
          frame True {
            n110 = control-ref of="Start Button"() -> (w144:refnum<vi>)
            n111 = property on="Property Node" class="Bool"(reference=w144, "DisabledEnum"=T18."Disabled and Grayed Out" ("Disabled")) -> ()  [unwired: 1 in, 2 out]
          }
        }
      }
      event Value Change {
        n112 = event-data() -> ("OldVal"=w151:refnum<visa-resource-name>)  [unwired: 1 in]
        n113 = local read "Settings Dialog"() -> (w152:T17)
        n114 = Unbundle By Name(w152) -> ("KNF SIMDOS Settings"=w149:T8)
        n115 = VISA Close(VISA resource name=w151) -> (error out=w150:errorcluster)  [unwired: 1 in]
        n116 = call "Initialize.vi"("error in (no error)"=w150, "KNF Settings In"=w149) -> ("No Pump Connected"=w148:bool)  [unwired: 6 in, 3 out]
        n117 = case shown="False" w148 {
          frame False {
            n118 = local read "Input Selected"() -> (w153:bool)
            n119 = case shown="True" w153 {
              frame False {
              }
              frame True {
                n120 = control-ref of="Start Button"() -> (w156:refnum<vi>)
                n121 = property on="Property Node" class="Bool"(reference=w156, "DisabledEnum"=T18."Enabled" ("Disabled")) -> ()  [unwired: 1 in, 2 out]
              }
            }
            n122 = local write "Output Selected"(TRUE) -> ()
          }
          frame True {
            n123 = control-ref of="Start Button"() -> (w157:refnum<vi>)
            n124 = property on="Property Node" class="Bool"(reference=w157, "DisabledEnum"=T18."Disabled and Grayed Out" ("Disabled")) -> ()  [unwired: 1 in, 2 out]
          }
        }
      }
      event Value Change {
        n125 = event-data() -> ("OldVal"=w165:refnum<visa-resource-name>)  [unwired: 1 in]
        n126 = local read "Settings Dialog"() -> (w166:T17)
        n127 = Unbundle By Name(w166) -> ("FLOM Settings"=w160:T10)
        n128 = VISA Close(VISA resource name=w165) -> (error out=w162:errorcluster)  [unwired: 1 in]
        n129 = Unbundle By Name(w160) -> ("Pump Number"=w159:dbl)
        n130 = case shown="Default" w159 {
          tunnel: w162 -> [w169 _]
          tunnel: [w168 FALSE ("Initialized")] -> w161
          tunnel: w160 -> [w167 _]
          frame Default {
            n131 = call "Initialize.vi"("error in (no error)"=w169, "FLOM Settings in"=w167) -> ("Initialized"=w168:bool)  [unwired: 6 in, 3 out]
          }
          frame 0 {
            n132 = One Button Dialog(message="Choose a Pump Number") -> ()  [unwired: 1 in, 1 out]
          }
        }
        n133 = case shown="True" w161 {
          frame False {
            n134 = control-ref of="Start Button"() -> (w172:refnum<vi>)
            n135 = property on="Property Node" class="Bool"(reference=w172, "DisabledEnum"=T18."Disabled and Grayed Out" ("Disabled")) -> ()  [unwired: 1 in, 2 out]
          }
          frame True {
            n136 = local read "Input Selected"() -> (w174:bool)
            n137 = case shown="True" w174 {
              frame False {
              }
              frame True {
                n138 = control-ref of="Start Button"() -> (w177:refnum<vi>)
                n139 = property on="Property Node" class="Bool"(reference=w177, "DisabledEnum"=T18."Enabled" ("Disabled")) -> ()  [unwired: 1 in, 2 out]
              }
            }
            n140 = local write "Output Selected"(TRUE) -> ()
          }
        }
      }
      event Value Change {
        n141 = event-data() -> ()  [unwired: 1 in, 1 out]
        n142 = local read "Settings Dialog"() -> (w183:T17)
        n143 = Unbundle By Name(w183) -> ("FLOM Settings"=w179:T10)
        n144 = Unbundle By Name(w179) -> ("Pump Number"=w178:dbl)
        n145 = case shown="Default" w178 {
          tunnel: [w185 FALSE ("Initialized")] -> w180
          tunnel: w179 -> [w184 _]
          frame Default {
            n146 = call "Initialize.vi"("FLOM Settings in"=w184) -> ("Initialized"=w185:bool)  [unwired: 7 in, 3 out]
          }
          frame 0 {
            n147 = One Button Dialog(message="Choose a non-zero Pump Number") -> ()  [unwired: 1 in, 1 out]
          }
        }
        n148 = case shown="True" w180 {
          frame False {
            n149 = control-ref of="Start Button"() -> (w188:refnum<vi>)
            n150 = property on="Property Node" class="Bool"(reference=w188, "DisabledEnum"=T18."Disabled and Grayed Out" ("Disabled")) -> ()  [unwired: 1 in, 2 out]
          }
          frame True {
            n151 = local read "Input Selected"() -> (w190:bool)
            n152 = case shown="True" w190 {
              frame False {
              }
              frame True {
                n153 = control-ref of="Start Button"() -> (w193:refnum<vi>)
                n154 = property on="Property Node" class="Bool"(reference=w193, "DisabledEnum"=T18."Enabled" ("Disabled")) -> ()  [unwired: 1 in, 2 out]
              }
            }
            n155 = local write "Output Selected"(TRUE) -> ()
          }
        }
      }
      event Value Change {
        n156 = event-data() -> ()  [unwired: 1 in, 1 out]
        n157 = local read "Settings Dialog"() -> (w198:T17)
        n158 = Unbundle By Name(w198) -> ("SSI PR Settings"=w194:T11)
        n159 = call "Initialize.vi"("SSI PR Settings In"=w194) -> ("Initialized"=w195:bool)  [unwired: 7 in, 3 out]
        n160 = case shown="True" w195 {
          frame False {
            n161 = control-ref of="Start Button"() -> (w199:refnum<vi>)
            n162 = property on="Property Node" class="Bool"(reference=w199, "DisabledEnum"=T18."Disabled and Grayed Out" ("Disabled")) -> ()  [unwired: 1 in, 2 out]
          }
          frame True {
            n163 = local read "Input Selected"() -> (w201:bool)
            n164 = case shown="True" w201 {
              frame False {
              }
              frame True {
                n165 = control-ref of="Start Button"() -> (w204:refnum<vi>)
                n166 = property on="Property Node" class="Bool"(reference=w204, "DisabledEnum"=T18."Enabled" ("Disabled")) -> ()  [unwired: 1 in, 2 out]
              }
            }
            n167 = local write "Output Selected"(TRUE) -> ()
          }
        }
      }
      event Value Change {
        n168 = event-data() -> ()  [unwired: 1 in, 6 out]
        n169 = local read "Input Selected"() -> (w205:bool)
        n170 = case shown="True" w205 {
          frame False {
          }
          frame True {
            n171 = control-ref of="Start Button"() -> (w210:refnum<vi>)
            n172 = property on="Property Node" class="Bool"(reference=w210, "DisabledEnum"=T18."Enabled" ("Disabled")) -> ()  [unwired: 1 in, 2 out]
          }
        }
        n173 = local write "Output Selected"(TRUE) -> ()
      }
      event Value Change {
        n174 = event-data() -> ("OldVal"=w214:refnum<visa-resource-name>)  [unwired: 1 in]
        n175 = local read "Settings Dialog"() -> (w217:T17)
        n176 = Unbundle By Name(w217) -> ("Bronkhorst M13 Flow Meter"=w216:T4)
        n177 = VISA Close(VISA resource name=w214) -> (error out=w215:errorcluster)  [unwired: 1 in]
        n178 = call "Initialize.vi"("error in (no error)"=w215, "Bronkhorst Settings in"=w216) -> ("No Meter Connnected"=w213:bool)  [unwired: 7 in, 2 out]
        n179 = case shown="False" w213 {
          frame False {
            n180 = local read "Output Selected"() -> (w218:bool)
            n181 = case shown="True" w218 {
              frame False {
              }
              frame True {
                n182 = control-ref of="Start Button"() -> (w221:refnum<vi>)
                n183 = property on="Property Node" class="Bool"(reference=w221, "DisabledEnum"=T18."Enabled" ("Disabled")) -> ()  [unwired: 1 in, 2 out]
              }
            }
            "Input Selected" <- TRUE ("Input Selected")
          }
          frame True {
            n184 = control-ref of="Start Button"() -> (w223:refnum<vi>)
            n185 = property on="Property Node" class="Bool"(reference=w223, "DisabledEnum"=T18."Disabled and Grayed Out" ("Disabled")) -> ()  [unwired: 1 in, 2 out]
            n186 = local write "Input Selected"(FALSE ("Input Selected")) -> ()
          }
        }
      }
      event Value Change {
        n187 = event-data() -> ("OldVal"=w228:refnum<visa-resource-name>)  [unwired: 1 in]
        n188 = local read "Settings Dialog"() -> (w231:T17)
        n189 = Unbundle By Name(w231) -> ("Bronkhorst M14 Settings"=w230:T13)
        n190 = VISA Close(VISA resource name=w228) -> (error out=w229:errorcluster)  [unwired: 1 in]
        n191 = call "Initialize.vi"("error in (no error)"=w229, "Bronkhorst Settings in"=w230) -> ("No Meter Connected"=w227:bool)  [unwired: 7 in, 2 out]
        n192 = case shown="False" w227 {
          frame False {
            n193 = local read "Output Selected"() -> (w232:bool)
            n194 = case shown="True" w232 {
              frame False {
              }
              frame True {
                n195 = control-ref of="Start Button"() -> (w235:refnum<vi>)
                n196 = property on="Property Node" class="Bool"(reference=w235, "DisabledEnum"=T18."Enabled" ("Disabled")) -> ()  [unwired: 1 in, 2 out]
              }
            }
            n197 = local write "Input Selected"(TRUE ("Input Selected")) -> ()
          }
          frame True {
            n198 = property on="Start Button" class="Bool"("DisabledEnum"=T18."Disabled and Grayed Out" ("Disabled")) -> ()  [unwired: 2 in, 2 out]
            n199 = local write "Input Selected"(FALSE ("Input Selected")) -> ()
          }
        }
      }
      event Value Change {
        n200 = event-data() -> ("NewVal"=w242:T5)  [unwired: 1 in]
        n201 = case "Show the correct settings" shown="\"Bronkhorst M13\"" w242 {
          tunnel: w239 -> [w245 w251 _]
          tunnel: [165.0 ("Data Entry Limits:Maximum") 1660.0 ("Data Entry Limits:Maximum") inf] -> w238
          frame "Bronkhorst M13" {
            n202 = Unbundle By Name(w245) -> ("Settings.Bronkhorst M13 Settings.VISA resource name"=w246:refnum<visa-resource-name>)
            n203 = control-ref of="VISA resource name"() -> (w247:refnum<vi>)
            n204 = property on="Bronkhorst M14 Settings" class="Clust (strict)"("Visible"=FALSE) -> ()  [unwired: 2 in, 2 out]
            n205 = property on="Bronkhorst M13 Flow Meter" class="Clust (strict)"("Visible"=TRUE) -> ()  [unwired: 2 in, 2 out]
            n206 = property on="Property Node" class="VISAName"(reference=w247, "Value"=w246) -> ()  [unwired: 1 in, 2 out]
          }
          frame "Bronkhorst M14" {
            n207 = Unbundle By Name(w251) -> ("Settings.Ismatech.VISA resource name"=w252:refnum<visa-resource-name>)
            n208 = control-ref of="VISA resource name"() -> (w253:refnum<vi>)
            n209 = property on="Bronkhorst M14 Settings" class="Clust (strict)"("Visible"=TRUE) -> ()  [unwired: 2 in, 2 out]
            n210 = property on="Bronkhorst M13 Flow Meter" class="Clust (strict)"("Visible"=FALSE) -> ()  [unwired: 2 in, 2 out]
            n211 = property on="Property Node" class="VISAName"(reference=w253, "Value"=w252) -> ()  [unwired: 1 in, 2 out]
          }
          frame "Default", Default {
            n212 = property on="Bronkhorst M13 Flow Meter" class="Clust (strict)"("Visible"=FALSE) -> ()  [unwired: 2 in, 2 out]
            n213 = property on="Bronkhorst M14 Settings" class="Clust (strict)"("Visible"=FALSE) -> ()  [unwired: 2 in, 2 out]
          }
        }
        n214 = property on="Maximum (ml/min)" class="DigNum (strict)"("Maximum"=w238) -> ()  [unwired: 2 in, 2 out]
      }
      event Value Change {
        n215 = event-data() -> ("NewVal"=w261:T6)  [unwired: 1 in]
        n216 = case "Show the correct settings" shown="\"Ismatec ISM 4308\"" w261 {
          tunnel: w258 -> [w269 w281 w293 w305 w318 _ _ _ w354 _]
          frame "Ismatec ISM 831C" {
            n217 = Unbundle By Name(w269) -> ("Settings.Ismatech.VISA resource name"=w270:refnum<visa-resource-name>)
            n218 = property on="VICI M50 Settings" class="Clust (strict)"("Visible"=FALSE) -> ()  [unwired: 2 in, 2 out]
            n219 = property on="Masterflex" class="Clust (strict)"("Visible"=FALSE) -> ()  [unwired: 2 in, 2 out]
            n220 = control-ref of="VISA resource name"() -> (w271:refnum<vi>)
            n221 = property on="Ismatech" class="Clust (strict)"("Visible"=TRUE) -> ()  [unwired: 2 in, 2 out]
            n222 = property on="FLOM Settings" class="Clust (strict)"("Visible"=FALSE) -> ()  [unwired: 2 in, 2 out]
            n223 = property on="Property Node" class="VISAName"(reference=w271, "Value"=w270) -> ()  [unwired: 1 in, 2 out]
            n224 = property on="KNF SIMDOS Settings" class="Clust (strict)"("Visible"=FALSE) -> ()  [unwired: 2 in, 2 out]
            n225 = property on="Tacmina Settings" class="Clust (strict)"("Visible"=FALSE) -> ()  [unwired: 2 in, 2 out]
            n226 = property on="Masterflex 75211 Settings" class="Clust (strict)"("Visible"=FALSE) -> ()  [unwired: 2 in, 2 out]
            n227 = property on="Ismatech 4308 Settings" class="Clust (strict)"("Visible"=FALSE) -> ()  [unwired: 2 in, 2 out]
            n228 = property on="SSI PR Settings" class="Clust (strict)"("Visible"=FALSE) -> ()  [unwired: 2 in, 2 out]
          }
          frame "Ismatec ISM 4308" {
            n229 = property on="VICI M50 Settings" class="Clust (strict)"("Visible"=FALSE) -> ()  [unwired: 2 in, 2 out]
            n230 = property on="Masterflex" class="Clust (strict)"("Visible"=FALSE) -> ()  [unwired: 2 in, 2 out]
            n231 = Unbundle By Name(w281) -> ("Settings.Ismatech 4308 Settings.VISA resource name"=w282:refnum<visa-resource-name>)
            n232 = control-ref of="VISA resource name"() -> (w283:refnum<vi>)
            n233 = property on="Ismatech" class="Clust (strict)"("Visible"=FALSE) -> ()  [unwired: 2 in, 2 out]
            n234 = property on="FLOM Settings" class="Clust (strict)"("Visible"=FALSE) -> ()  [unwired: 2 in, 2 out]
            n235 = property on="Property Node" class="VISAName"(reference=w283, "Value"=w282) -> ()  [unwired: 1 in, 2 out]
            n236 = property on="KNF SIMDOS Settings" class="Clust (strict)"("Visible"=FALSE) -> ()  [unwired: 2 in, 2 out]
            n237 = property on="Tacmina Settings" class="Clust (strict)"("Visible"=FALSE) -> ()  [unwired: 2 in, 2 out]
            n238 = property on="Masterflex 75211 Settings" class="Clust (strict)"("Visible"=FALSE) -> ()  [unwired: 2 in, 2 out]
            n239 = property on="Ismatech 4308 Settings" class="Clust (strict)"("Visible"=TRUE) -> ()  [unwired: 2 in, 2 out]
            n240 = property on="SSI PR Settings" class="Clust (strict)"("Visible"=FALSE) -> ()  [unwired: 2 in, 2 out]
          }
          frame "FLOM UI-22-11" {
            n241 = Unbundle By Name(w293) -> ("Settings.FLOM Settings.VISA resource name"=w294:refnum<visa-resource-name>)
            n242 = property on="Ismatech" class="Clust (strict)"("Visible"=FALSE) -> ()  [unwired: 2 in, 2 out]
            n243 = property on="FLOM Settings" class="Clust (strict)"("Visible"=TRUE) -> ()  [unwired: 2 in, 2 out]
            n244 = property on="VICI M50 Settings" class="Clust (strict)"("Visible"=FALSE) -> ()  [unwired: 2 in, 2 out]
            n245 = property on="Masterflex" class="Clust (strict)"("Visible"=FALSE) -> ()  [unwired: 2 in, 2 out]
            n246 = control-ref of="VISA resource name"() -> (w295:refnum<vi>)
            n247 = property on="Property Node" class="VISAName"(reference=w295, "Value"=w294) -> ()  [unwired: 1 in, 2 out]
            n248 = property on="Tacmina Settings" class="Clust (strict)"("Visible"=FALSE) -> ()  [unwired: 2 in, 2 out]
            n249 = property on="KNF SIMDOS Settings" class="Clust (strict)"("Visible"=FALSE) -> ()  [unwired: 2 in, 2 out]
            n250 = property on="Ismatech 4308 Settings" class="Clust (strict)"("Visible"=FALSE) -> ()  [unwired: 2 in, 2 out]
            n251 = property on="Masterflex 75211 Settings" class="Clust (strict)"("Visible"=FALSE) -> ()  [unwired: 2 in, 2 out]
            n252 = property on="SSI PR Settings" class="Clust (strict)"("Visible"=FALSE) -> ()  [unwired: 2 in, 2 out]
          }
          frame "Masterflex 7550-30" {
            n253 = Unbundle By Name(w305) -> ("Settings.Masterflex.VISA resource name"=w306:refnum<visa-resource-name>)
            n254 = control-ref of="VISA resource name"() -> (w307:refnum<vi>)
            n255 = property on="Ismatech" class="Clust (strict)"("Visible"=FALSE) -> ()  [unwired: 2 in, 2 out]
            n256 = property on="FLOM Settings" class="Clust (strict)"("Visible"=FALSE) -> ()  [unwired: 2 in, 2 out]
            n257 = property on="VICI M50 Settings" class="Clust (strict)"("Visible"=FALSE) -> ()  [unwired: 2 in, 2 out]
            n258 = property on="Masterflex" class="Clust (strict)"("Visible"=TRUE) -> ()  [unwired: 2 in, 2 out]
            n259 = property on="Property Node" class="VISAName"(reference=w307, "Value"=w306) -> ()  [unwired: 1 in, 2 out]
            n260 = property on="Tacmina Settings" class="Clust (strict)"("Visible"=FALSE) -> ()  [unwired: 2 in, 2 out]
            n261 = property on="KNF SIMDOS Settings" class="Clust (strict)"("Visible"=FALSE) -> ()  [unwired: 2 in, 2 out]
            n262 = property on="Masterflex 75211 Settings" class="Clust (strict)"("Visible"=FALSE) -> ()  [unwired: 2 in, 2 out]
            n263 = property on="Ismatech 4308 Settings" class="Clust (strict)"("Visible"=FALSE) -> ()  [unwired: 2 in, 2 out]
            n264 = property on="SSI PR Settings" class="Clust (strict)"("Visible"=FALSE) -> ()  [unwired: 2 in, 2 out]
          }
          frame "VICI M6" {
            n265 = Unbundle By Name(w318) -> ("Settings.VICI M50 Settings.VISA resource name"=w317:refnum<visa-resource-name>)
            n266 = property on="Ismatech" class="Clust (strict)"("Visible"=FALSE) -> ()  [unwired: 2 in, 2 out]
            n267 = property on="FLOM Settings" class="Clust (strict)"("Visible"=FALSE) -> ()  [unwired: 2 in, 2 out]
            n268 = property on="VICI M50 Settings" class="Clust (strict)"("Visible"=TRUE) -> ()  [unwired: 2 in, 2 out]
            n269 = property on="Masterflex" class="Clust (strict)"("Visible"=FALSE) -> ()  [unwired: 2 in, 2 out]
            n270 = property on="VISA resource name" class="VISAName"("Value"=w317) -> ()  [unwired: 2 in, 2 out]
            n271 = property on="KNF SIMDOS Settings" class="Clust (strict)"("Visible"=FALSE) -> ()  [unwired: 2 in, 2 out]
            n272 = property on="Tacmina Settings" class="Clust (strict)"("Visible"=FALSE) -> ()  [unwired: 2 in, 2 out]
            n273 = property on="Masterflex 75211 Settings" class="Clust (strict)"("Visible"=FALSE) -> ()  [unwired: 2 in, 2 out]
            n274 = property on="Ismatech 4308 Settings" class="Clust (strict)"("Visible"=FALSE) -> ()  [unwired: 2 in, 2 out]
            n275 = property on="SSI PR Settings" class="Clust (strict)"("Visible"=FALSE) -> ()  [unwired: 2 in, 2 out]
          }
          frame "Default", Default {
            n276 = property on="KNF SIMDOS Settings" class="Clust (strict)"("Visible"=FALSE) -> ()  [unwired: 2 in, 2 out]
            n277 = property on="FLOM Settings" class="Clust (strict)"("Visible"=FALSE) -> ()  [unwired: 2 in, 2 out]
            n278 = property on="Masterflex" class="Clust (strict)"("Visible"=FALSE) -> ()  [unwired: 2 in, 2 out]
            n279 = property on="Tacmina Settings" class="Clust (strict)"("Visible"=FALSE) -> ()  [unwired: 2 in, 2 out]
            n280 = property on="VICI M50 Settings" class="Clust (strict)"("Visible"=FALSE) -> ()  [unwired: 2 in, 2 out]
            n281 = property on="Ismatech" class="Clust (strict)"("Visible"=FALSE) -> ()  [unwired: 2 in, 2 out]
            n282 = property on="Masterflex 75211 Settings" class="Clust (strict)"("Visible"=FALSE) -> ()  [unwired: 2 in, 2 out]
            n283 = property on="Ismatech 4308 Settings" class="Clust (strict)"("Visible"=FALSE) -> ()  [unwired: 2 in, 2 out]
            n284 = property on="SSI PR Settings" class="Clust (strict)"("Visible"=FALSE) -> ()  [unwired: 2 in, 2 out]
          }
          frame "Tacmina QI" {
            n285 = property on="FLOM Settings" class="Clust (strict)"("Visible"=FALSE) -> ()  [unwired: 2 in, 2 out]
            n286 = property on="KNF SIMDOS Settings" class="Clust (strict)"("Visible"=FALSE) -> ()  [unwired: 2 in, 2 out]
            n287 = property on="Tacmina Settings" class="Clust (strict)"("Visible"=TRUE) -> ()  [unwired: 2 in, 2 out]
            n288 = property on="Ismatech" class="Clust (strict)"("Visible"=FALSE) -> ()  [unwired: 2 in, 2 out]
            n289 = property on="Masterflex" class="Clust (strict)"("Visible"=FALSE) -> ()  [unwired: 2 in, 2 out]
            n290 = property on="VICI M50 Settings" class="Clust (strict)"("Visible"=FALSE) -> ()  [unwired: 2 in, 2 out]
            n291 = property on="Ismatech 4308 Settings" class="Clust (strict)"("Visible"=FALSE) -> ()  [unwired: 2 in, 2 out]
            n292 = property on="Masterflex 75211 Settings" class="Clust (strict)"("Visible"=FALSE) -> ()  [unwired: 2 in, 2 out]
            n293 = property on="SSI PR Settings" class="Clust (strict)"("Visible"=FALSE) -> ()  [unwired: 2 in, 2 out]
          }
          frame "SSI PR/LD" {
            n294 = property on="FLOM Settings" class="Clust (strict)"("Visible"=FALSE) -> ()  [unwired: 2 in, 2 out]
            n295 = property on="KNF SIMDOS Settings" class="Clust (strict)"("Visible"=FALSE) -> ()  [unwired: 2 in, 2 out]
            n296 = property on="Tacmina Settings" class="Clust (strict)"("Visible"=FALSE) -> ()  [unwired: 2 in, 2 out]
            n297 = property on="Ismatech" class="Clust (strict)"("Visible"=FALSE) -> ()  [unwired: 2 in, 2 out]
            n298 = property on="Masterflex" class="Clust (strict)"("Visible"=FALSE) -> ()  [unwired: 2 in, 2 out]
            n299 = property on="VICI M50 Settings" class="Clust (strict)"("Visible"=FALSE) -> ()  [unwired: 2 in, 2 out]
            n300 = property on="Ismatech 4308 Settings" class="Clust (strict)"("Visible"=FALSE) -> ()  [unwired: 2 in, 2 out]
            n301 = property on="Masterflex 75211 Settings" class="Clust (strict)"("Visible"=FALSE) -> ()  [unwired: 2 in, 2 out]
            n302 = property on="SSI PR Settings" class="Clust (strict)"("Visible"=TRUE) -> ()  [unwired: 2 in, 2 out]
          }
          frame "KNF SIMDOS" {
            n303 = Unbundle By Name(w354) -> ("Settings.KNF SIMDOS Settings.VISA resource name"=w355:refnum<visa-resource-name>)
            n304 = property on="Ismatech" class="Clust (strict)"("Visible"=FALSE) -> ()  [unwired: 2 in, 2 out]
            n305 = property on="FLOM Settings" class="Clust (strict)"("Visible"=FALSE) -> ()  [unwired: 2 in, 2 out]
            n306 = property on="VICI M50 Settings" class="Clust (strict)"("Visible"=FALSE) -> ()  [unwired: 2 in, 2 out]
            n307 = property on="Masterflex" class="Clust (strict)"("Visible"=FALSE) -> ()  [unwired: 2 in, 2 out]
            n308 = property on="VISA resource name" class="VISAName"("Value"=w355) -> ()  [unwired: 2 in, 2 out]
            n309 = property on="Tacmina Settings" class="Clust (strict)"("Visible"=FALSE) -> ()  [unwired: 2 in, 2 out]
            n310 = property on="KNF SIMDOS Settings" class="Clust (strict)"("Visible"=TRUE) -> ()  [unwired: 2 in, 2 out]
            n311 = property on="Ismatech 4308 Settings" class="Clust (strict)"("Visible"=FALSE) -> ()  [unwired: 2 in, 2 out]
            n312 = property on="Masterflex 75211 Settings" class="Clust (strict)"("Visible"=FALSE) -> ()  [unwired: 2 in, 2 out]
            n313 = property on="SSI PR Settings" class="Clust (strict)"("Visible"=FALSE) -> ()  [unwired: 2 in, 2 out]
          }
          frame "Masterflex 75211-70" {
            n314 = property on="FLOM Settings" class="Clust (strict)"("Visible"=FALSE) -> ()  [unwired: 2 in, 2 out]
            n315 = property on="KNF SIMDOS Settings" class="Clust (strict)"("Visible"=FALSE) -> ()  [unwired: 2 in, 2 out]
            n316 = property on="Tacmina Settings" class="Clust (strict)"("Visible"=FALSE) -> ()  [unwired: 2 in, 2 out]
            n317 = property on="Ismatech" class="Clust (strict)"("Visible"=FALSE) -> ()  [unwired: 2 in, 2 out]
            n318 = property on="Masterflex" class="Clust (strict)"("Visible"=FALSE) -> ()  [unwired: 2 in, 2 out]
            n319 = property on="VICI M50 Settings" class="Clust (strict)"("Visible"=FALSE) -> ()  [unwired: 2 in, 2 out]
            n320 = property on="Masterflex 75211 Settings" class="Clust (strict)"("Visible"=TRUE) -> ()  [unwired: 2 in, 2 out]
            n321 = property on="Ismatech 4308 Settings" class="Clust (strict)"("Visible"=FALSE) -> ()  [unwired: 2 in, 2 out]
            n322 = property on="SSI PR Settings" class="Clust (strict)"("Visible"=FALSE) -> ()  [unwired: 2 in, 2 out]
          }
        }
      }
      event "Cancel Button": Value Change; Panel Close {
        # "True: Stop While Loop and Close Dialog"
        n323 = event-data() -> ()  [unwired: 1 in, 1 out]
        n324 = call-poly "Enqueue Message.vi"("Message"="Exit", "Message Queue"=w370) -> ()  [unwired: 8 in, 2 out]
        n325 = call "Generate Temporary Report.vi"("Line of Events"=string[] ["Canceled"], "Module Name"=w368) -> ()  [unwired: 9 in, 1 out]
      }
      event "Accept Button": Value Change {
        # "True: Stop While Loop and Close Dialog"
        n326 = event-data() -> ()  [unwired: 1 in, 1 out]
        n327 = call-poly "Enqueue Message.vi"("Message"="Accept", "Message Queue"=w377) -> ()  [unwired: 8 in, 2 out]
        n328 = call "Generate Temporary Report.vi"("Line of Events"=string[] ["Accepted"], "Module Name"=w375) -> ()  [unwired: 9 in, 1 out]
      }
      event "Decline Button": Value Change {
        # "True: Stop While Loop and Close Dialog"
        n329 = event-data() -> ()  [unwired: 1 in, 1 out]
        n330 = call-poly "Enqueue Message.vi"("Message"="Decline", "Message Queue"=w384) -> ()  [unwired: 8 in, 2 out]
        n331 = call "Generate Temporary Report.vi"("Line of Events"=string[] ["Declined"], "Module Name"=w382) -> ()  [unwired: 9 in, 1 out]
      }
    }
  }
  n332 = timed-loop {
    tunnel: w15 -> [w413]
    shift-right: [w391] -> w12
    shift-left: w14 -> [w410]
    tunnel: [w409] -> w2
    tunnel: w13 -> [w407]
    shift-right: [w405] -> _
    shift-left: w8 -> [w404]
    timing: w11 -> [_]
    timing-out: [_] -> w10
    shift-right: [w403] -> _
    shift-left: w8 -> [w402]
    shift-right: [w401] -> _
    shift-left: _ -> [w400]
    shift-right: [w399] -> _
    shift-left: 0 -> [w398]
    shift-right: [w397] -> _
    shift-left: w8 -> [w396]
    shift-right: [w395] -> _
    shift-left: w8 -> [w394]
    shift-right: [w393] -> _
    shift-left: _ -> [w392]
    tunnel: [w390] -> w7
    tunnel: w1 -> [w389]
    stop <- w408 stop-if-true
    n333 = node-c288() -> ()  [unwired: 1 in]
    n334 = call "Dequeue Message.vi"("error in (no error)"=w407, "Message Queue"=w413) -> ("error out"=w406:errorcluster, "Message Data"=w412:variant, "Message"=w411:string, "dup Message Queue"=w390:refnum<queue>)  [unwired: 6 in]
    n335 = case shown="\"Calculate\"" w411 {
      tunnel: w410 -> [w424 w456 w495 w524 w629 w656 w679 w839 w849]
      tunnel: w412 -> [_ _ _ _ _ _ _ _ _]
      tunnel: [w424 w425 w510 w532 w625 w656 w679 w839 w844] -> w391
      tunnel: [w423 w467 w498 w533 w614 w657 w677 w825 w850] -> w409
      tunnel: w406 -> [w423 w467 w511 _ w628 w657 w685 w829 w851]
      tunnel: [_ _ _ _ FALSE FALSE FALSE FALSE TRUE] -> w408
      tunnel: w390 -> [_ _ w512 w536 _ _ w686 w831 _]
      tunnel: [w422 w466 w492 w541 w616 w650 w691 w835 w848] -> w405
      tunnel: w404 -> [w422 w466 _ w541 w616 w650 w691 w835 w848]
      tunnel: [w421 w465 w504 w548 w640 w655 w694 w838 w847] -> w403
      tunnel: w402 -> [w421 w465 w504 w547 w640 w655 w694 w838 w847]
      tunnel: [w420 w464 w505 w544 w639 w654 w693 w837 w846] -> w401
      tunnel: w400 -> [w420 w464 _ w543 w639 w654 w693 w837 w846]
      tunnel: w398 -> [w419 w463 w503 w539 w633 w648 w689 w833 w845]
      tunnel: [w419 w463 w503 w537 w633 w648 w689 w833 w845] -> w399
      tunnel: [w418 w462 w502 w530 w631 w651 w692 w836 w843] -> w397
      tunnel: w396 -> [w418 w462 w502 w529 w631 w651 w692 w836 w843]
      tunnel: [w417 w461 w501 w528 w636 w649 w690 w834 w842] -> w395
      tunnel: w394 -> [w417 w461 w501 w527 w636 w649 w690 w834 w842]
      tunnel: [w416 w460 w500 w526 w632 w647 w688 w832 w841] -> w393
      tunnel: w392 -> [w416 w460 w500 w525 w632 w647 w688 w832 w841]
      tunnel: w389 -> [_ _ _ _ w615 _ _ _ _]
      frame Default {
      }
      frame "Start Pressed" {
        w455 = T18."Disabled and Grayed Out" ("Disabled")
        # "Close the old connections"
        n336 = Unbundle By Name(w456) -> ("Settings.PID 2 Parameters.Input Device"=w457:T5, "Settings.PID 2 Parameters.Output Device"=w458:T6)
        n337 = Unbundle By Name("Settings Dialog") -> ("Ismatech"=w440:T2, "Ismatech 4308 Settings"=w430:T12, "Masterflex"=w441:T3, "Bronkhorst M13 Flow Meter"=w442:T4, "Setup Parameters"=w443:cluster{"Input Device":T5, "Output Device":T6}, "Bronkhorst M14 Settings"=w446:T13, "Tacmina Settings"=w447:T7, "KNF SIMDOS Settings"=w438:T8, "VICI M50 Settings"=w439:T9, "FLOM Settings"=w449:T10, "SSI PR Settings"=w437:T11, "Calibration Limits.Steps"=w452:dbl, "Calibration Limits"=w453:T26, "File Name"=w454:string)
        n338 = case shown="\"Default\", Default" w458 {
          tunnel: w456 -> [_ w475 w477 w479 _ w482]
          frame "Default", Default {
          }
          frame "Ismatec ISM 831C" {
            n339 = Unbundle By Name(w475) -> ("Settings.Ismatech.VISA resource name"=w476:refnum<visa-resource-name>)
            n340 = VISA Close(VISA resource name=w476) -> ()  [unwired: 1 in, 1 out]
          }
          frame "Masterflex 7550-30" {
            n341 = Unbundle By Name(w477) -> ("Settings.Masterflex.VISA resource name"=w478:refnum<visa-resource-name>)
            n342 = VISA Close(VISA resource name=w478) -> ()  [unwired: 1 in, 1 out]
          }
          frame "VICI M6" {
            n343 = Unbundle By Name(w479) -> ("Settings.Ismatech.VISA resource name"=w480:refnum<visa-resource-name>)
            n344 = VISA Close(VISA resource name=w480) -> ()  [unwired: 1 in, 1 out]
          }
          frame "Tacmina QI" {
            # "No VISA to Close"
          }
          frame "KNF SIMDOS" {
            n345 = Unbundle By Name(w482) -> ("Settings.KNF SIMDOS Settings.VISA resource name"=w481:refnum<visa-resource-name>)
            n346 = VISA Close(VISA resource name=w481) -> ()  [unwired: 1 in, 1 out]
          }
        }
        n347 = Unbundle(w443) -> ("Input Device"=w444:T5, "Output Device"=w445:T6)
        n348 = case shown="\"KNF SIMDOS\"" w445 {
          tunnel: w438 -> [w472 w473]
          tunnel: [w471 w474] -> w448
          frame "Default", Default {
            n349 = Unbundle(w472) -> ("VISA resource name"=w469:refnum<visa-resource-name>, "Simulated?"=w468:bool)
            n350 = Bundle(cluster=T8 {"VISA resource name"="", "Simulated?"=TRUE} ("KNF Settings"), "VISA resource name"=w469, "Simulated?"=w468) -> (w471:T8)
          }
          frame "KNF SIMDOS" {
            n351 = call "Initialize.vi"("KNF Settings In"=w473) -> ("KNF Settings Out"=w474:T8)  [unwired: 7 in, 3 out]
          }
        }
        n352 = Concatenate Strings(w454, " Calibration Data %Y-%m-%dT%H.%M.%S.csv" ("time format string (%c)")) -> (w435:string)
        n353 = Format Date/Time String(time format string (%c)=w435) -> (date/time string=w433:string)  [unwired: 2 in]
        n354 = Build Path(base path=path "C:/Users/Public/Documents/Calibration Data", name or relative path=w433) -> (appended path=w432:path)
        n355 = Open/Create/Replace File(file path (use dialog)=w432, operation (0:open)=T23."open or create") -> (refnum out=w451:refnum<file>)  [unwired: 4 in, 2 out]
        n356 = case shown="\"Default\", Default" w457 {
          tunnel: w456 -> [_ w484 w485 w487]
          frame "Default", Default {
          }
          frame "Bronkhorst M13" {
            n357 = Unbundle By Name(w484) -> ("Settings.Bronkhorst M13 Settings.VISA resource name"=w483:refnum<visa-resource-name>)
            n358 = VISA Close(VISA resource name=w483) -> ()  [unwired: 1 in, 1 out]
          }
          frame "Bronkhorst M14" {
            n359 = Unbundle By Name(w485) -> ("Settings.Ismatech.VISA resource name"=w486:refnum<visa-resource-name>)
            n360 = VISA Close(VISA resource name=w486) -> ()  [unwired: 1 in, 1 out]
          }
          frame "Scale Rate of Change" {
            n361 = Unbundle By Name(w487) -> ("Settings.Ismatech.VISA resource name"=w488:refnum<visa-resource-name>)
            n362 = VISA Close(VISA resource name=w488) -> ()  [unwired: 1 in, 1 out]
          }
        }
        n363 = Bundle By Name(cluster=w456, "Settings.Cycle Period"=500.0, "Settings.Ismatech"=w440, "Settings.Ismatech 4308 Settings"=w430, "Settings.Masterflex"=w441, "Settings.Bronkhorst M13 Settings"=w442, "Settings.PID 2 Parameters.Input Device"=w444, "Settings.PID 2 Parameters.Output Device"=w445, "Settings.Bronkhorst M14 Settings"=w446, "Settings.Tacmina Settings"=w447, "Settings.KNF SIMDOS Settings"=w448, "Settings.VICI M50 Settings"=w439, "Settings.FLOM Settings"=w449, "Settings.SSI PR Settings"=w437, "File Refnum"=w451, "Settings.Calibration Limits.Steps"=w452, "Settings.Calibration Limits"=w453) -> (w425:T1)
        n364 = property on="Cancel Button" class="Bool"("DisabledEnum"=w455) -> ()  [unwired: 2 in, 2 out]
        n365 = property on="Start Button" class="Bool"("DisabledEnum"=w455) -> ()  [unwired: 2 in, 2 out]
        n366 = Variant To Flattened String(Variant=w425) -> (data string=w428:string)  [unwired: 1 out]
        n367 = Build Array (concatenate)(string[] ["Calibration Settings Updated "] ("Line of Events"), w428) -> (w427:string[])
        n368 = call "Generate Temporary Report.vi"("Line of Events"=w427, "Module Name"="Calibration") -> ()  [unwired: 9 in, 1 out]
      }
      frame "Initialize" {
        n369 = call "Initialize.vi"("error in"=w511, "Pump Calibration Config in"=w495) -> ("error out"=w499:errorcluster, "Pump Calibration Config Out"=w510:T1)  [unwired: 8 in]
        n370 = Unbundle By Name(w495) -> ("Settings.Calibration Limits"=w509:T26)
        n371 = Unbundle By Name(w509) -> ("Minimum (ml/min)"=w493:dbl, "Maximum (ml/min)"=w491:dbl, "Steps"=w490:dbl)
        n372 = Subtract(x=w491, y=w493) -> (x-y=w508:dbl)
        n373 = Subtract(x=w490, y=2.0) -> (x-y=w496:dbl)
        n374 = Decrement(x=w490) -> (x-1=w489:dbl)
        n375 = Divide(x=w508, y=w489) -> (x/y=w506:dbl)
        n376 = for {
          N: w496 -> [_]
          tunnel: w493 -> [w517]
          tunnel: w506 -> [w516]
          tunnel: dbl[] [] -> [w519]
          tunnel: [w518] -> w494 mode=concatenating
          i -> [w515]
          n377 = Increment(x=w515) -> (x+1=w514:i32)
          n378 = Multiply(x=w516, y=w514) -> (x*y=w521:dbl)
          n379 = Add(x=w517, y=w521) -> (x+y=w520:dbl)
          n380 = Build Array (concatenate)(w519, w520) -> (w518:dbl[])
        }
        n381 = Build Array (concatenate)(w493, w494, w491) -> (w492:dbl[])
        "Step Array" <- w492
        n382 = Get Date/Time In Seconds() -> (seconds since 1Jan1904=w505:timestamp)
        n383 = call-poly "Enqueue Message.vi"("error in (no error)"=w499, "Message"="Run", "Message Queue"=w512) -> ("error out"=w498:errorcluster)  [unwired: 7 in, 1 out]
      }
      frame "Run" {
        n384 = Get Date/Time In Seconds() -> (seconds since 1Jan1904=w535:timestamp)
        n385 = Subtract(x=w535, y=w543) -> (x-y=w546:dbl)
        n386 = call "Input.vi"("Pump Calibration Config in"=w524) -> ("error out"=w549:errorcluster, "Pump Calibration Config Out"=w523:T1)  [unwired: 9 in]
        n387 = Greater?(x=w546, y=30.0) -> (0:w542:bool)
        n388 = case shown="False" w542 {
          tunnel: w523 -> [w568 w585]
          tunnel: [w569 w590] -> w548
          tunnel: w547 -> [w570 w590]
          tunnel: [w567 w593] -> w544
          tunnel: w543 -> [w567 _]
          tunnel: w541 -> [w566 w581]
          tunnel: w539 -> [w565 w576]
          tunnel: [w561 w579] -> w538
          tunnel: [w565 w575] -> w537
          tunnel: w536 -> [w564 w586]
          tunnel: w535 -> [w559 _]
          tunnel: [w552 w580] -> w530
          tunnel: w529 -> [w552 w583]
          tunnel: [w551 w577] -> w528
          tunnel: w527 -> [w551 w578]
          tunnel: [w550 w573] -> w526
          tunnel: w525 -> [w550 _]
          frame False {
            w555 = "," ("string")
            n389 = Unbundle By Name(w568) -> ("Flowmeter Output"=w560:dbl, "File Refnum"=w563:refnum<file>)
            n390 = call-poly "Enqueue Message.vi"("Message"="Run", "Message Queue"=w564) -> ()  [unwired: 8 in, 2 out]
            n391 = Index Array(array=w566, index=w565) -> (element=w561:dbl)
            n392 = Number To Fractional String(number=w560) -> (F-format string=w554:string)  [unwired: 3 in]
            n393 = Number To Fractional String(number=w561) -> (F-format string=w556:string)  [unwired: 3 in]
            n394 = Get Date/Time String(seconds (now)=w559) -> (time string=w557:string)  [unwired: 2 in, 1 out]
            n395 = Concatenate Strings(w557, w555, w556, w555, w554, "\r\n") -> (w562:string)
            n396 = Write to Text File(file (use dialog)=w563, text=w562) -> ()  [unwired: 2 in, 3 out]
            n397 = Build Array (concatenate)(w570, w560) -> (w569:dbl[])
          }
          frame True {
            w587 = 15 ("y")
            n398 = Unbundle By Name(w585) -> ("Settings.Calibration Limits.Steps"=w571:dbl)
            n399 = Index Array(array=w581, index=w576) -> (element=w579:dbl)
            n400 = Array Size(array=w590) -> (size(s)=w592:i32)
            n401 = Decrement(x=w571) -> (x-1=w572:dbl)
            n402 = Equal?(x=w576, y=w572) -> (x = y?=w584:bool)
            n403 = Subtract(x=w592, y=w587) -> (x-y=w591:i32)
            n404 = case shown="False" w584 {
              tunnel: w586 -> [w596 w600]
              tunnel: w576 -> [w595 w599]
              tunnel: [w594 w599] -> w575
              frame False {
                n405 = Increment(x=w595) -> (x+1=w594:i32)
                n406 = call-poly "Enqueue Message.vi"("Message"="Run", "Message Queue"=w596) -> ()  [unwired: 8 in, 2 out]
              }
              frame True {
                n407 = call-poly "Enqueue Message.vi"("Message"="Calculate", "Message Queue"=w600) -> ()  [unwired: 8 in, 2 out]
              }
            }
            n408 = Array Subset(array=w590, index=w591) -> (w589:dbl[])  [unwired: 1 in]
            n409 = Add Array Elements(numeric array=w589) -> (sum=w588:dbl)
            n410 = Divide(x=w588, y=w587) -> (x/y=w582:dbl)
            n411 = Build Array (concatenate)(w578, w579) -> (w577:dbl[])
            "X array" <- w577
            n412 = Build Array (concatenate)(w583, w582) -> (w580:dbl[])
            "Y array" <- w580
            n413 = Bundle(w577, w580) -> (w574:cluster{dbl[], dbl[]})  [unwired: 1 in]
            n414 = Build Array(w574) -> (w573:cluster{dbl[], dbl[]}[])
            n415 = local write "Calibration Graph"(w573) -> ()
            n416 = Get Date/Time In Seconds() -> (seconds since 1Jan1904=w593:timestamp)
          }
        }
        n417 = Bundle By Name(cluster=w523, "Speed %"=w538) -> (w540:T1)
        n418 = call "Output.vi"("error in (no error)"=w549, "Pump Calibration Config in"=w540) -> ("error out"=w534:errorcluster, "Pump Calibration Config Out"=w522:T1)  [unwired: 8 in]
        n419 = call "Pump Status.vi"("error in (no error)"=w534, "Pump Calibration Config in"=w522) -> ("error out"=w533:errorcluster, "Pump Calibration Config out"=w532:T1)  [unwired: 8 in]
        n420 = Unbundle By Name(w532) -> ("Pump On?"=→"Pump Status":enum16{"Off", "On", "Not Initialized"})
      }
      frame "Calculate" {
        w619 = "," ("string")
        n421 = call <vilib>:"Linear Fit.vi"("Y"=w631, "X"=w616, "parameter bounds"=T25 {"slope min"=-inf, "slope max"=inf, "intercept min"=-inf, "intercept max"=inf}) -> ("Best Linear Fit"=w630:dbl[], "slope"=w609:dbl, "intercept"=w608:dbl)  [unwired: 8 in, 2 out]
        "Calibration Slope" <- w609
        "Y Intercept" <- w608
        n422 = for {
          tunnel: w616 -> [w645] mode=indexing
          tunnel: w609 -> [w644]
          tunnel: w608 -> [w643]
          tunnel: [w642] -> w617 mode=indexing
          workers-P: _ -> [_]
          n423 = Multiply(x=w645, y=w644) -> (x*y=w646:dbl)
          n424 = Add(x=w646, y=w643) -> (x+y=w642:dbl)
        }
        n425 = call <vilib>:"Goodness of Fit.vi"("Best Fit"=w630, "Y"=w631) -> ("R-square"=w610:dbl)  [unwired: 6 in, 3 out]
        "R^2 Value" <- w610
        n426 = call "Close.vi"("error in (no error)"=w628, "Pump Calibration Config in"=w629) -> ("error out"=w626:errorcluster, "Pump Calibration Config out"=w627:T1)  [unwired: 8 in]
        n427 = Number To Fractional String(number=w609) -> (F-format string=w622:string)  [unwired: 3 in]
        n428 = Number To Fractional String(number=w610) -> (F-format string=w621:string)  [unwired: 3 in]
        n429 = Number To Fractional String(number=w608) -> (F-format string=w618:string)  [unwired: 3 in]
        n430 = call "Pump Status.vi"("error in (no error)"=w626, "Pump Calibration Config in"=w627) -> ("error out"=w613:errorcluster, "Pump Calibration Config out"=w625:T1)  [unwired: 8 in]
        n431 = Concatenate Strings(w619, w619, w619, w622, w619, w621, w619, w618, "\r\n") -> (w623:string)
        n432 = Unbundle By Name(w625) -> ("File Refnum"=w624:refnum<file>)
        n433 = Bundle(w616, w617) -> (w634:cluster{dbl[], dbl[]})  [unwired: 1 in]
        n434 = Bundle(w616, w631) -> (w637:cluster{dbl[], dbl[]})  [unwired: 1 in]
        n435 = Write to Text File(file (use dialog)=w624, text=w623) -> ()  [unwired: 2 in, 3 out]
        n436 = Build Array(w637, w634) -> (→"Calibration Graph":cluster{dbl[], dbl[]}[])
        n437 = Bundle By Name(cluster=T24 {"R^2"=0.0, "Calibration Slope"=0.0, "Y Intercept"=0.0}, "R^2"=w610, "Calibration Slope"=w609, "Y Intercept"=w608) -> (w607:T24)
        n438 = Flatten To XML(anything=w607) -> (xml string=w602:string)
        n439 = Search and Replace String(replace all?=TRUE ("replace all? (F)"), input string=w602, search string="\r\n", replace string="_" ("replace string (\"\")")) -> (result string=w601:string)  [unwired: 4 in, 3 out]
        n440 = Build Array (concatenate)(string[] ["Calculated Final Values"] ("Line of Events"), w601) -> (w606:string[])
        n441 = call "Generate Temporary Report.vi"("error in (no error)"=w613, "Line of Events"=w606, "Module Name"=w615) -> ("error out"=w614:errorcluster)  [unwired: 8 in]
      }
      frame "Close File" {
        n442 = Unbundle By Name(w656) -> ("File Refnum"=w653:refnum<file>)
        n443 = Not A Number/Path/Refnum?(number/path/refnum=w653) -> (NaN/Path/Refnum?=w652:bool)
        n444 = case shown="False" w652 {
          tunnel: w653 -> [w659 _]
          frame False {
            n445 = Close File(refnum=w659) -> ()  [unwired: 1 in, 2 out]
          }
          frame True {
          }
        }
      }
      frame "Accept" {
        w662 = "," ("string")
        w672 = path "C:/Users/Public/Documents/Calibration Data/Pumps Calibration Curves.csv" ("Pump Module Config.Settings.Pump Calibration File")
        n446 = call-poly "Enqueue Message.vi"("error in (no error)"=w685, "Message"="Close File", "Message Queue"=w686) -> ("error out"=w682:errorcluster, "dup Message Queue"=w683:refnum<queue>)  [unwired: 7 in]
        n447 = property on="Calibration Slope" class="DigNum (strict)"() -> ("Value"=w678:dbl)  [unwired: 2 in, 2 out]
        n448 = call-poly "Enqueue Message.vi"("error in (no error)"=w682, "Message"="Exit", "Message Queue"=w683) -> ("error out"=w676:errorcluster)  [unwired: 7 in, 1 out]
        n449 = call-poly <vilib>:"Read Delimited Spreadsheet.vi"("file path (dialog if empty)"=w672, "delimiter (\\t)"="\n" ("delimiter (\\t)")) -> ("all rows"=w666:string[][])  [unwired: 8 in, 5 out]
        n450 = property on="Y Intercept" class="DigNum (strict)"() -> ("Value"=w661:dbl)  [unwired: 2 in, 2 out]
        n451 = property on="File Name" class="Str"(error in=w676) -> (error out=w671:errorcluster, "Text.Text"=w669:string)  [unwired: 1 in, 1 out]
        n452 = Number To Fractional String(number=w678) -> (F-format string=w668:string)  [unwired: 3 in]
        n453 = Number To Fractional String(number=w661) -> (F-format string=w660:string)  [unwired: 3 in]
        n454 = for {
          tunnel: w669 -> [w703]
          tunnel: w666 -> [w702] mode=indexing
          tunnel: [w697] -> w665
          tunnel: [w696] -> w663
          i -> [w696]
          stop <- w697 stop-if-true
          n455 = Index Array(array=w702, index=0) -> (element=w699:string)
          n456 = xnode "Match Regular Expression"("input string"=w699, "regular expression"="^([^,])+") -> ("whole match"=w698:string)  [unwired: 4 in, 4 out]
          n457 = Equal?(x=w698, y=w703) -> (x = y?=w697:bool)
        }
        n458 = Concatenate Strings(w669, w662, w668, w662, w660) -> (w667:string)
        n459 = Open/Create/Replace File(file path (use dialog)=w672, error in=w671, operation (0:open)=T23."replace or create") -> (error out=w670:errorcluster)  [unwired: 3 in, 2 out]
        n460 = Build Array(w667) -> (w664:string[])
        n461 = case shown="False" w665 {
          tunnel: w666 -> [w819 w824]
          tunnel: w663 -> [_ w823]
          tunnel: [w818 w822] -> w674
          tunnel: w664 -> [w820 w821]
          frame False {
            n462 = Build Array (concatenate)(w819, w820) -> (w818:string[][])
          }
          frame True {
            n463 = Replace Array Subset(array=w824, new element=w821, index (row)=w823) -> (w822:string[][])  [unwired: 1 in]
          }
        }
        n464 = call-poly <vilib>:"Write Delimited Spreadsheet.vi"("file path (dialog if empty)"=w672, "2D data"=w674, "append to file? (new file:F)"=TRUE, "error in (no error)"=w670, "delimiter (\\t)"="," ("delimiter (\\t)")) -> ("error out"=w677:errorcluster)  [unwired: 9 in, 1 out]
      }
      frame "Decline" {
        n465 = call-poly "Enqueue Message.vi"("error in (no error)"=w829, "Message"="Close File", "Message Queue"=w831) -> ("error out"=w826:errorcluster, "dup Message Queue"=w827:refnum<queue>)  [unwired: 7 in]
        n466 = call-poly "Enqueue Message.vi"("error in (no error)"=w826, "Message"="Exit", "Message Queue"=w827) -> ("error out"=w825:errorcluster)  [unwired: 7 in, 1 out]
      }
      frame "Exit" {
        n467 = call "Close.vi"("error in (no error)"=w851, "Pump Calibration Config in"=w849) -> ("error out"=w850:errorcluster, "Pump Calibration Config out"=w844:T1)  [unwired: 8 in]
      }
    }
    n468 = node-c288() -> ()  [unwired: 1 in, 1 out]
  }
  "error out" <- w2
  "Pump Calibration Config out" <- w12
  n469 = node-c288(w10) -> ()  [unwired: 1 out]
  n470 = Release Queue(queue=w7) -> ()  [unwired: 2 in, 3 out]
  n471 = Variant To Flattened String(Variant=w2) -> (data string=w5:string)  [unwired: 1 out]
  n472 = Build Array (concatenate)(string[] ["Collect any Errors on Program Closure "] ("Line of Events"), w5) -> (w4:string[])
  n473 = call "Generate Temporary Report.vi"("Line of Events"=w4, "Module Name"="Calibration") -> ()  [unwired: 9 in, 1 out]
